vi "CSMsettings_ut_test.vi"(8 "Error In":errorcluster, 11 "CSMinfo in":T3={"Общие сведения"={"Регистрационный номер заказа"="", "Идентификация (шифр) образца"="", "IMEI образца"="", "НД, устанавливающий требования"="", "Методы испытаний (измерений)"="", "Дата начала испытаний"="", "Дата завершения испытаний"=""}, "Климатические условия внешней среды"={"Температура окружающего воздуха"="", "Относительная влажность воздуха"="", "Атмосферное давление"=""}, "Окно с настройками"={"Режим звонка связь"=0, "Напряжение источника"=0, "Условия окружающей среды"=0, "Номер образца"=0, "Источник питания"=0, "Номер испытания"=0, "Режим звонка тональный модем"=0, "Количество итераций TM"=100.0, "Аутентификация"=0, "Колличество повторов измерений"=1.0, "Сим карта"=0, "VISA adress of CMW500"="", "Input attenuation"=1.0, "Output attenuation"=1.0, "Call Release Type"=0, "GSM Band"=0, "BCCH Channel Number"=0.0, "TCH Channel Number"=0.0, "Codec"=0, "AWGN"=0, "snrRatioInDb"=0.0, "GSM Fading"=0, "UL C/I ratio"=0, "Use a custom network ID"=FALSE, "MCC (Mobile Country Code)"=0.0, "MNC (Mobile Network Code)"=0.0, "NCC (Network Color Code)"=0.0, "MNC digit count"=0, "BCC (Base station Color Code)"=0.0, "LAC (Location Area Code)"=0.0, "RAC (Routing Area Code)"=0.0, "Cell Identity"=0.0, "Override UE ID"=FALSE, "MCC (UE Mobile Country Code)"=0.0, "MNC (UE Mobile Network Code)"=0.0, "MSIN (Mobile Subscription ID)"=0.0, "InputScaleFactor"=0, "OutputScaleFactor"=0, "Post MSD wave file playback 3GPP  26.269 \nEU_DTMF_tones"=FALSE, "Scenario"=0, "AlAckBehavior"=0, "PSAP listens for PUSH"=FALSE, "BCCH Channel Power"=0.0, "TCH Channel Power"=0.0, "Setting Path"=path "", "Алгоритм дозвона"=0}} {"Окно с настройками"."Алгоритм дозвона" items=["Standart", "Recall"]; "Окно с настройками"."AlAckBehavior" items=["POSITIVE", "CLEAR_DOWN", "LOOP_BACK_MSD_PART"]; "Окно с настройками"."Scenario" items=["NORMAL", "NORMAL_IMMEDIATE_START", "TIMEOUT_T3", "ALLRV_REQ", "SUPPRESS_MSD", "SUPPRESS_ALACK", "SUPPRESS_SEND_MSD"]; "Окно с настройками"."OutputScaleFactor" items=["ONE", "QUARTER", "HALF", "TWO", "FOUR"]; "Окно с настройками"."InputScaleFactor" items=["ONE", "QUARTER", "HALF", "TWO", "FOUR"]; "Окно с настройками"."MNC digit count" items=["TWO", "THREE"]; "Окно с настройками"."UL C/I ratio" items=["Ci1Db", "Ci4Db", "Ci7Db", "Ci10Db", "Ci13Db", "Ci16Db"]; "Окно с настройками"."GSM Fading" items=["GsmFadingOff", "GsmEtsiTs103412DlFading", "GsmEtsiTs103412UlFading", "GsmEtsiTs103412DlUlFading"]; "Окно с настройками"."AWGN" items=["Off", "50MhzAwgn"]; "Окно с настройками"."Codec" items=["FRV2", "AMRH_GMSK_7K95", "AMRH_GMSK_7K40", "AMRH_GMSK_6K70", "AMRH_GMSK_5K90", "AMRH_GMSK_5K15", "AMRH_GMSK_4K75", "AMRF_GMSK_12K20", "AMRF_GMSK_10K20", "AMRF_GMSK_7K95", "AMRF_GMSK_7K40 ", "AMRF_GMSK_6K70", "AMRF_GMSK_5K90", "AMRF_GMSK_5K15", "AMRF_GMSK_4K75", "FRV1", "HRV1", "WAMR_GMSK_6K60", "WAMR_GMSK_8K85", "WAMR_GMSK_12K65"]; "Окно с настройками"."GSM Band" items=["GSM450", "GSM850", "GSM900", "GSM1800", "GSM1900"]; "Окно с настройками"."Call Release Type" items=["NormalRelease", "CallInterruption"]; "Окно с настройками"."Сим карта" items=["SIM", "eSIM"]; "Окно с настройками"."Колличество повторов измерений" min=1.0 max=100.0 format="%#_3g"; "Окно с настройками"."Аутентификация" items=["On", "Off"]; "Окно с настройками"."Режим звонка тональный модем" items=["Автоматически (AT) GEMALTO", "Автоматически (AT) SIMCOM", "Автоматически (AT) SIMCOM SIM7600E-H", "Автоматически (AT) TELIT", "Автоматически (AT) PROGRESS", "Автоматически (AT) PROGRESS GREEN", "Автоматически (AT) PROGRESS BLUE", "Автоматически (реле)", "Вручную"]; "Окно с настройками"."Номер испытания" items=["1", "2", "3"]; "Окно с настройками"."Источник питания" items=["Не используется", "IT6332A"]; "Окно с настройками"."Номер образца" items=["1", "2", "3"]; "Окно с настройками"."Условия окружающей среды" items=["UnormTnorm", "UminTmin", "UmaxTmin", "UminTmax", "UmaxTmax", "TypeA", "TypeB"]; "Окно с настройками"."Напряжение источника" items=["12", "24"]; "Окно с настройками"."Режим звонка связь" items=["Автоматически (AT) GEMALTO", "Автоматически (AT) SIMCOM", "Автоматически (AT) SIMCOM SIM7600E-H", "Автоматически (AT) TELIT", "Автоматически (AT) PROGRESS", "Автоматически (AT) PROGRESS GREEN", "Автоматически (AT) PROGRESS BLUE", "Автоматически (реле)", "Вручную"]}) -> (0 "Error Out":errorcluster, 3 "CSMinfo out":T3={"Общие сведения"={"Регистрационный номер заказа"="", "Идентификация (шифр) образца"="", "IMEI образца"="", "НД, устанавливающий требования"="", "Методы испытаний (измерений)"="", "Дата начала испытаний"="", "Дата завершения испытаний"=""}, "Климатические условия внешней среды"={"Температура окружающего воздуха"="", "Относительная влажность воздуха"="", "Атмосферное давление"=""}, "Окно с настройками"={"Режим звонка связь"=0, "Напряжение источника"=0, "Условия окружающей среды"=0, "Номер образца"=0, "Источник питания"=0, "Номер испытания"=0, "Режим звонка тональный модем"=0, "Количество итераций TM"=0.0, "Аутентификация"=0, "Колличество повторов измерений"=1.0, "Сим карта"=0, "VISA adress of CMW500"="", "Input attenuation"=1.0, "Output attenuation"=1.0, "Call Release Type"=0, "GSM Band"=0, "BCCH Channel Number"=0.0, "TCH Channel Number"=0.0, "Codec"=0, "AWGN"=0, "snrRatioInDb"=0.0, "GSM Fading"=0, "UL C/I ratio"=0, "Use a custom network ID"=FALSE, "MCC (Mobile Country Code)"=0.0, "MNC (Mobile Network Code)"=0.0, "NCC (Network Color Code)"=0.0, "MNC digit count"=0, "BCC (Base station Color Code)"=0.0, "LAC (Location Area Code)"=0.0, "RAC (Routing Area Code)"=0.0, "Cell Identity"=0.0, "Override UE ID"=FALSE, "MCC (UE Mobile Country Code)"=0.0, "MNC (UE Mobile Network Code)"=0.0, "MSIN (Mobile Subscription ID)"=0.0, "InputScaleFactor"=0, "OutputScaleFactor"=0, "Post MSD wave file playback 3GPP  26.269 \nEU_DTMF_tones"=FALSE, "Scenario"=0, "AlAckBehavior"=0, "PSAP listens for PUSH"=FALSE, "BCCH Channel Power"=0.0, "TCH Channel Power"=0.0, "Setting Path"=path "", "Алгоритм дозвона"=0}} {"Окно с настройками"."Алгоритм дозвона" items=["Standart", "Recall"]; "Окно с настройками"."AlAckBehavior" items=["POSITIVE", "CLEAR_DOWN", "LOOP_BACK_MSD_PART"]; "Окно с настройками"."Scenario" items=["NORMAL", "NORMAL_IMMEDIATE_START", "TIMEOUT_T3", "ALLRV_REQ", "SUPPRESS_MSD", "SUPPRESS_ALACK", "SUPPRESS_SEND_MSD"]; "Окно с настройками"."OutputScaleFactor" items=["ONE", "QUARTER", "HALF", "TWO", "FOUR"]; "Окно с настройками"."InputScaleFactor" items=["ONE", "QUARTER", "HALF", "TWO", "FOUR"]; "Окно с настройками"."MNC digit count" items=["TWO", "THREE"]; "Окно с настройками"."UL C/I ratio" items=["Ci1Db", "Ci4Db", "Ci7Db", "Ci10Db", "Ci13Db", "Ci16Db"]; "Окно с настройками"."GSM Fading" items=["GsmFadingOff", "GsmEtsiTs103412DlFading", "GsmEtsiTs103412UlFading", "GsmEtsiTs103412DlUlFading"]; "Окно с настройками"."AWGN" items=["Off", "50MhzAwgn"]; "Окно с настройками"."Codec" items=["FRV2", "AMRH_GMSK_7K95", "AMRH_GMSK_7K40", "AMRH_GMSK_6K70", "AMRH_GMSK_5K90", "AMRH_GMSK_5K15", "AMRH_GMSK_4K75", "AMRF_GMSK_12K20", "AMRF_GMSK_10K20", "AMRF_GMSK_7K95", "AMRF_GMSK_7K40 ", "AMRF_GMSK_6K70", "AMRF_GMSK_5K90", "AMRF_GMSK_5K15", "AMRF_GMSK_4K75", "FRV1", "HRV1", "WAMR_GMSK_6K60", "WAMR_GMSK_8K85", "WAMR_GMSK_12K65"]; "Окно с настройками"."GSM Band" items=["GSM450", "GSM850", "GSM900", "GSM1800", "GSM1900"]; "Окно с настройками"."Call Release Type" items=["NormalRelease", "CallInterruption"]; "Окно с настройками"."Сим карта" items=["SIM", "eSIM"]; "Окно с настройками"."Колличество повторов измерений" min=1.0 max=100.0 format="%#_3g"; "Окно с настройками"."Аутентификация" items=["On", "Off"]; "Окно с настройками"."Режим звонка тональный модем" items=["Автоматически (AT) GEMALTO", "Автоматически (AT) SIMCOM", "Автоматически (AT) SIMCOM SIM7600E-H", "Автоматически (AT) TELIT", "Автоматически (AT) PROGRESS", "Автоматически (AT) PROGRESS GREEN", "Автоматически (AT) PROGRESS BLUE", "Автоматически (реле)", "Вручную"]; "Окно с настройками"."Номер испытания" items=["1", "2", "3"]; "Окно с настройками"."Источник питания" items=["Не используется", "IT6332A"]; "Окно с настройками"."Номер образца" items=["1", "2", "3"]; "Окно с настройками"."Условия окружающей среды" items=["UnormTnorm", "UminTmin", "UmaxTmin", "UminTmax", "UmaxTmax", "TypeA", "TypeB"]; "Окно с настройками"."Напряжение источника" items=["12", "24"]; "Окно с настройками"."Режим звонка связь" items=["Автоматически (AT) GEMALTO", "Автоматически (AT) SIMCOM", "Автоматически (AT) SIMCOM SIM7600E-H", "Автоматически (AT) TELIT", "Автоматически (AT) PROGRESS", "Автоматически (AT) PROGRESS GREEN", "Автоматически (AT) PROGRESS BLUE", "Автоматически (реле)", "Вручную"]})   [LabVIEW 2018]
uses:
  CSMinfo.ctl
  MOKO_LabViewLibrary/MokoSTM/MokoClassicUtilitySTM/MCUS_STM.ctl
  MOKO_LabViewLibrary/MokoSTM/MokoClassicUtilitySTM/MCUS_ITEM.ctl
  <vilib>/addons/_JKI.lib/Serialization/JSON/JKI JSON Serialization.lvlib
panel:
  in  "Reset":bool
  in  "Open":bool
  in  "Save":bool
  in  "Setting Path":path
  in  "Применить":bool
  in  "Общие настройки/Настройки модема":T1(tab)
  in  "Алгоритм дозвона":u16(ring) items=["Standart", "Recall"]
  in  "Сим карта":u16(ring) items=["SIM", "eSIM"]
  in  "Количество повторов измерений":dbl=1.0
  in  "Аунтетификация":u16(ring) items=["On", "Off"]
  in  "Количество итераций TM":dbl=100.0
  in  "Условия окружающей среды":u16(ring) items=["UnormTnorm", "UminTmin", "UmaxTmin", "UminTmax", "UmaxTmax", "TypeA", "TypeB"]
  in  "Режим звонка тональный модем":u16(ring) items=["Автоматически (AT) GEMALTO", "Автоматически (AT) SIMCOM", "Автоматически (AT) SIMCOM SIM7600E-H", "Автоматически (AT) TELIT", "Автоматически (AT) PROGRESS", "Автоматически (AT) PROGRESS GREEN", "Автоматически (AT) PROGRESS BLUE", "Автоматически (реле)", "Вручную"]
  in  "Номер испытания":u16(ring) items=["1", "2", "3"]
  in  "Источник питания":u16(ring) items=["Не используется", "IT6332A"]
  in  "Напряжение источника":u16(ring) items=["12", "24"]
  in  "Номер образца":u16(ring) items=["1", "2", "3"]
  in  "Режим звонка связь":u16(ring) items=["Автоматически (AT) GEMALTO", "Автоматически (AT) SIMCOM", "Автоматически (AT) SIMCOM SIM7600E-H", "Автоматически (AT) TELIT", "Автоматически (AT) PROGRESS", "Автоматически (AT) PROGRESS GREEN", "Автоматически (AT) PROGRESS BLUE", "Автоматически (реле)", "Вручную"]
  in  "Настройки модема по умолчанию":enum32{"CMW500", "GSM", "PSAP"}(tab)
  in  "VISA adress of CMW500":string="TCPIP0::169.254.98.10::inst0::INSTR"
  in  "Input attenuation":dbl=1.0
  in  "Output attenuation":dbl=100.0
  in  "GSM":T2(tab)
  in  "BCCH Channel Power":dbl=1.0
  in  "TCH Channel Power":dbl=1.0
  in  "GSM Band":u16(ring) items=["GSM450", "GSM850", "GSM900", "GSM1800", "GSM1900"]
  in  "BCCH Channel Number":dbl=1.0
  in  "TCH Channel number":dbl=1.0
  in  "Codec":u16(ring) items=["FRV2", "AMRH_GMSK_7K95", "AMRH_GMSK_7K40", "AMRH_GMSK_6K70", "AMRH_GMSK_5K90", "AMRH_GMSK_5K15", "AMRH_GMSK_4K75", "AMRF_GMSK_12K20", "AMRF_GMSK_10K20", "AMRF_GMSK_7K95", "AMRF_GMSK_7K40 ", "AMRF_GMSK_6K70", "AMRF_GMSK_5K90", "AMRF_GMSK_5K15", "AMRF_GMSK_4K75", "FRV1", "HRV1", "WAMR_GMSK_6K60", "WAMR_GMSK_8K85", "WAMR_GMSK_12K65"]
  in  "AWGN":u16(ring) items=["Off", "50MhzAwgn"]
  in  "snrRatioInDb":dbl=1.0
  in  "GSM Fading":u16(ring) items=["GsmFadingOff", "GsmEtsiTs103412DlFading", "GsmEtsiTs103412UlFading", "GsmEtsiTs103412DlUlFading"]
  in  "UL C/I ratio":u16(ring) items=["Ci1Db", "Ci4Db", "Ci7Db", "Ci10Db", "Ci13Db", "Ci16Db"]
  in  "MCC (Mobile Country Code)":dbl=1.0
  in  "Use a custom network ID":bool
  in  "MNC (Mobile Network Code)":dbl=1.0
  in  "MNC digit count":u16(ring) items=["TWO", "THREE"]
  in  "BCC (Base station Color Code)":dbl=1.0
  in  "NCC (Network Color Code)":dbl=1.0
  in  "RAC (Routing Area Code)":dbl=1.0
  in  "LAC (Location Area Code)":dbl=1.0
  in  "Cell Identity":dbl=1.0
  in  "Override UE ID":bool
  in  "MNC (UE Mobile Network Code)":dbl=1.0
  in  "MCC (UE Mobile Country Code)":dbl=1.0
  in  "MSIN (Mobile Subscription ID)":dbl=1.0 format="%#_10g"
  in  "Call Release Type":u16(ring) items=["NormalRelease", "CallInterruption"]
  in  "OutputScaleFactor":u16(ring) items=["ONE", "QUARTER", "HALF", "TWO", "FOUR"]
  in  "PSAP listens for PUSH":bool
  in  "AlAckBehavior":u16(ring) items=["POSITIVE", "CLEAR_DOWN", "LOOP_BACK_MSD_PART"]
  in  "Scenario":u16(ring) items=["NORMAL", "NORMAL_IMMEDIATE_START", "TIMEOUT_T3", "ALLRV_REQ", "SUPPRESS_MSD", "SUPPRESS_ALACK", "SUPPRESS_SEND_MSD"]
  in  "InputScaleFactor":u16(ring) items=["ONE", "QUARTER", "HALF", "TWO", "FOUR"]
  in  "Post MSD wave file playback 3GPP  26.269 EU_DTMF_tones":bool
  # "0,4\n0,6\n1\n1,5\n1,6\n2,5\n4"
  # "kPa\nbar\nkgf/cm2\nMPa"
  # "1. Общие настройки"
  # "Номер образца:"
  # "Номер испытания:"
  # "Режим измерения:"
  # "Источник питания:"
  # "Напряжение источника питания, B:"
  # "2. Настройки связи"
  # "Режим звонка:"
  # "Аунтетификация:"
  # "Сим карта:"
  # "Количество повторов измерений:"
  # "3. Настройки тонального модема"
  # "Режим звонка:"
  # "Алгоритм дозвона:"
  # "Количество итераций Tonal:"
  # "VISA adress of CMW500:"
  # "Input attenuation:"
  # "Output attenuation:"
  # "GSM Band:"
  # "BCCH Channel Power"
  # "TCH Channel Power"
  # "BCCH Channel Number"
  # "TCH Channel number"
  # "Codec"
  # "8.6.6"
  # "AWGN"
  # "snrRatioInDb"
  # "GSM Fading"
  # "UL C/I ratio"
  # "MCC (Mobile Country Code)"
  # "MNC (Mobile Network Code)"
  # "MNC digit count"
  # "NCC (Network Color Code)"
  # "BCC (Base station Color Code)"
  # "LAC (Location Area Code)"
  # "RAC (Routing Area Code)"
  # "Cell Identity"
  # "MCC (UE Mobile Country Code)"
  # "MNC (UE Mobile Network Code)"
  # "MSIN (Mobile Subscription ID)"
  # "Call Release Type:"
  # "8.6.6"
  # "InputScaleFactor"
  # "OutputScaleFactor"
  # "8.6.7"
  # "8.6.8 (Use parameter NORMAL_IMMEDIATE_START)"
  # "Scenario"
  # "8.6.9 (Use parameter LOOP_BACK_MSD_PART)"
  # "AlAckBehavior"
  # "1. Общие настройки"
  # "Настройки модема по умолчанию"
  # "CMW500"
  # "PSAP"
  # "8.6.6"
  # "8.6.7"
  # "GSM"
  # "2. Настройки связи"
  # "8.6.8 (Use parameter NORMAL_IMMEDIATE_START)"
  # "8.6.9 (Use parameter LOOP_BACK_MSD_PART)"
  # "8.6.6"
  # "3. Настройки тонального модема"
  # "1. Общие настройки"
  # "Настройки модема по умолчанию"
  # "CMW500"
  # "PSAP"
  # "8.6.6"
  # "8.6.7"
  # "GSM"
  # "2. Настройки связи"
  # "8.6.8 (Use parameter NORMAL_IMMEDIATE_START)"
  # "8.6.9 (Use parameter LOOP_BACK_MSD_PART)"
  # "8.6.6"
  # "3. Настройки тонального модема"
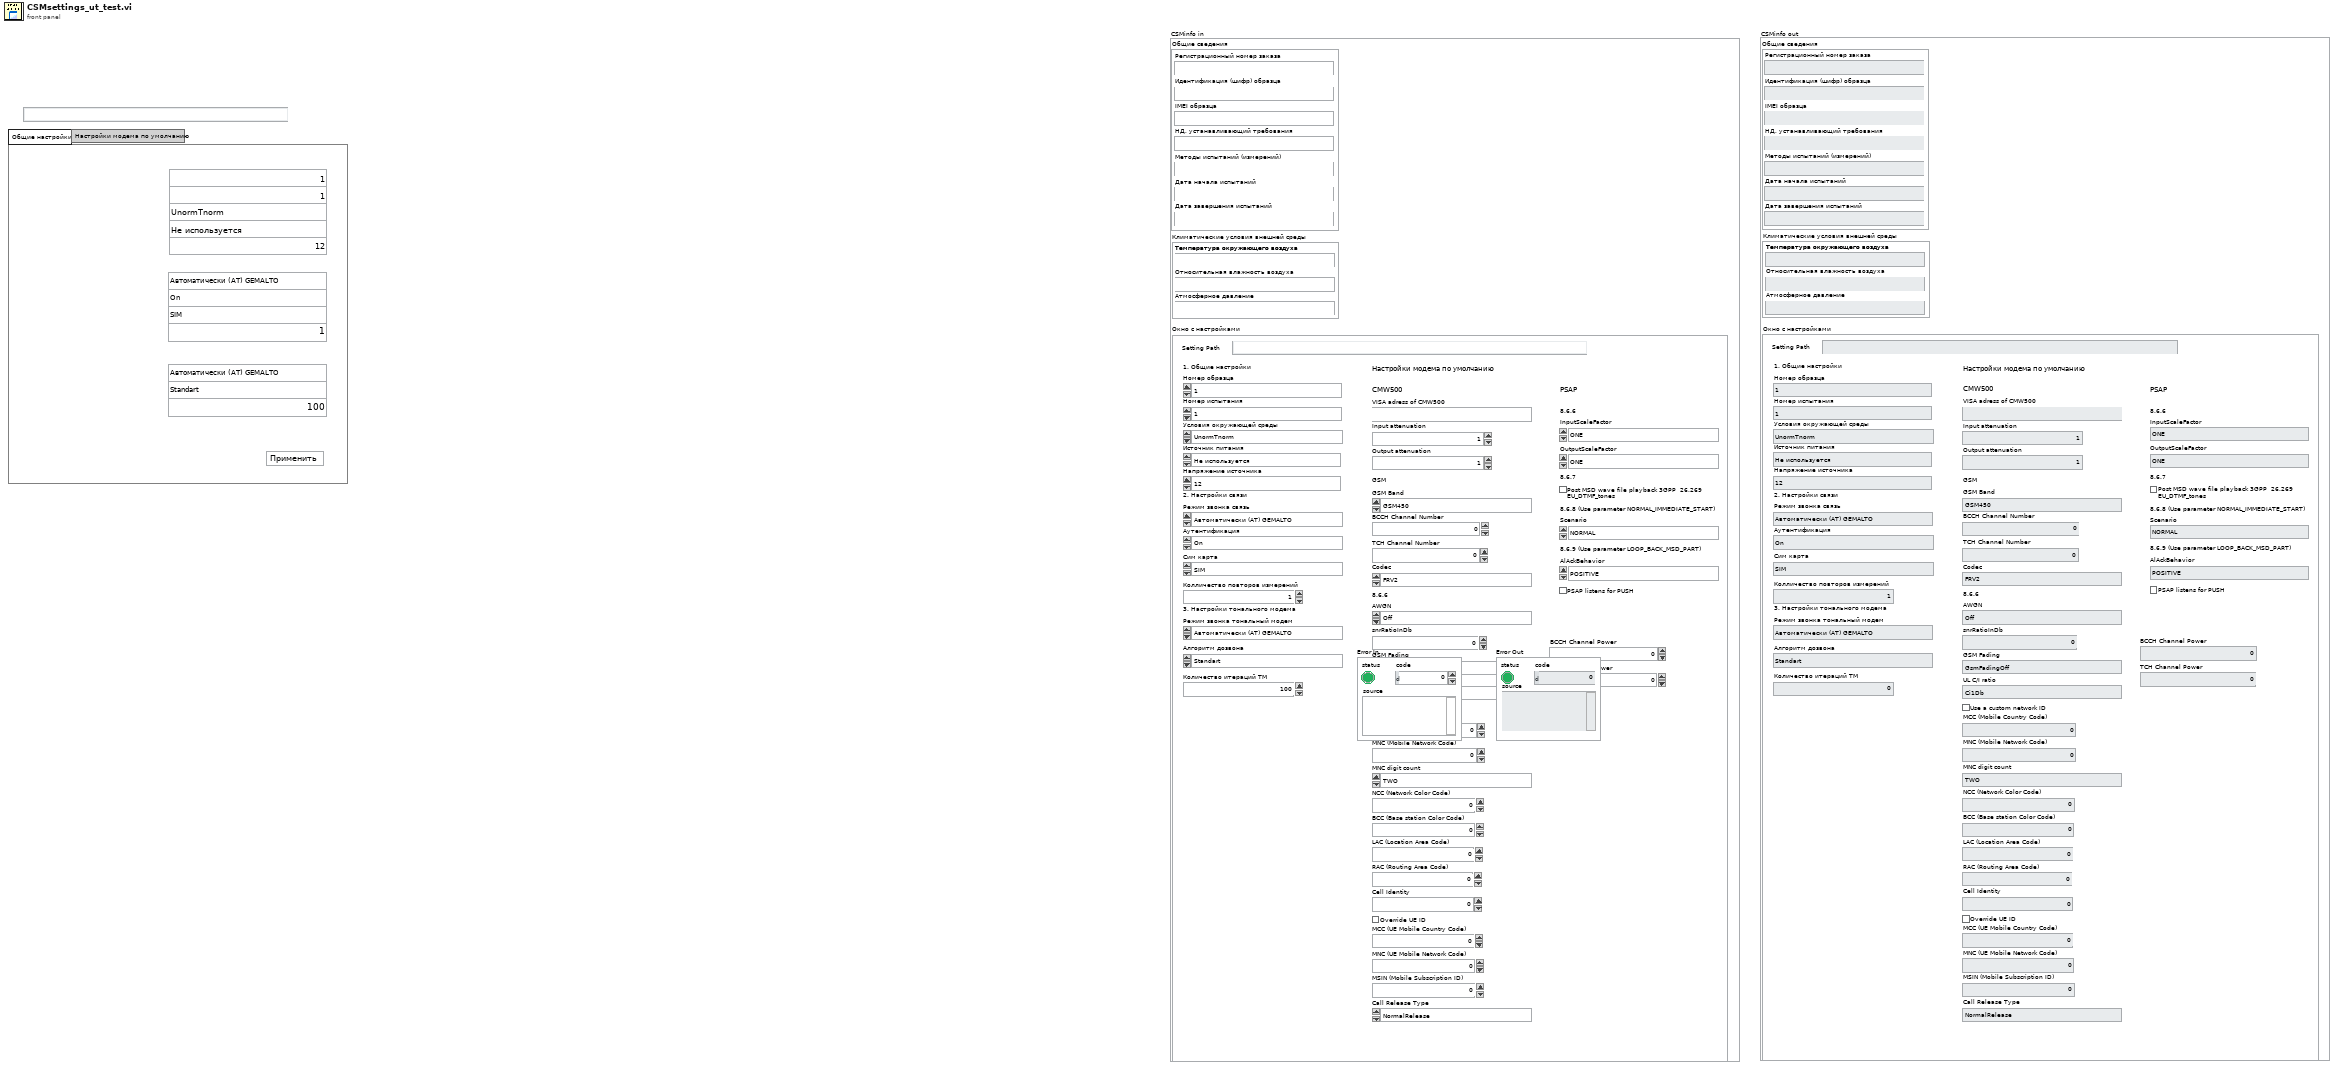
[diagram p1: front panel]
types:
  T1 = enum32{"Общие настройки", "Настройки модема по умолчанию"}
  T2 = enum32{"GSM Band/AWGN", "Custom network ID", "Call Release Type"}
  T3 = typedef "CSMinfo.ctl" = cluster{"Общие сведения":cluster{"Регистрационный номер заказа":string, "Идентификация (шифр) образца":string, "IMEI образца":string, "НД, устанавливающий требования":string, "Методы испытаний (измерений)":string, "Дата начала испытаний":string, "Дата завершения испытаний":string}, "Климатические условия внешней среды":cluster{"Температура окружающего воздуха":string, "Относительная влажность воздуха":string, "Атмосферное давление":string}, "Окно с настройками":cluster{"Режим звонка связь":u16, "Напряжение источника":u16, "Условия окружающей среды":u16, "Номер образца":u16, "Источник питания":u16, "Номер испытания":u16, "Режим звонка тональный модем":u16, "Количество итераций TM":dbl, "Аутентификация":u16, "Колличество повторов измерений":dbl, "Сим карта":u16, "VISA adress of CMW500":string, "Input attenuation":dbl, "Output attenuation":dbl, "Call Release Type":u16, "GSM Band":u16, "BCCH Channel Number":dbl, "TCH Channel Number":dbl, "Codec":u16, "AWGN":u16, "snrRatioInDb":dbl, "GSM Fading":u16, "UL C/I ratio":u16, "Use a custom network ID":bool, "MCC (Mobile Country Code)":dbl, "MNC (Mobile Network Code)":dbl, "NCC (Network Color Code)":dbl, "MNC digit count":u16, "BCC (Base station Color Code)":dbl, "LAC (Location Area Code)":dbl, "RAC (Routing Area Code)":dbl, "Cell Identity":dbl, "Override UE ID":bool, "MCC (UE Mobile Country Code)":dbl, "MNC (UE Mobile Network Code)":dbl, "MSIN (Mobile Subscription ID)":dbl, "InputScaleFactor":u16, "OutputScaleFactor":u16, "Post MSD wave file playback 3GPP  26.269 \nEU_DTMF_tones":bool, "Scenario":u16, "AlAckBehavior":u16, "PSAP listens for PUSH":bool, "BCCH Channel Power":dbl, "TCH Channel Power":dbl, "Setting Path":path, "Алгоритм дозвона":u16}}
  T4 = typedef "MCUS_STM.ctl" = cluster{"main stm":T5, "data":string}
  T5 = typedef "MCUS_ITEM.ctl" = enum16{"idle", "_____ main_____ ", "Init", "Stop", "Apply values", "Save", "Open", "Reset"}
  T6 = cluster{"Режим звонка связь":u16, "Напряжение источника":u16, "Условия окружающей среды":u16, "Номер образца":u16, "Источник питания":u16, "Номер испытания":u16, "Режим звонка тональный модем":u16, "Количество итераций TM":dbl, "Аутентификация":u16, "Колличество повторов измерений":dbl, "Сим карта":u16, "VISA adress of CMW500":string, "Input attenuation":dbl, "Output attenuation":dbl, "Call Release Type":u16, "GSM Band":u16, "BCCH Channel Number":dbl, "TCH Channel Number":dbl, "Codec":u16, "AWGN":u16, "snrRatioInDb":dbl, "GSM Fading":u16, "UL C/I ratio":u16, "Use a custom network ID":bool, "MCC (Mobile Country Code)":dbl, "MNC (Mobile Network Code)":dbl, "NCC (Network Color Code)":dbl, "MNC digit count":u16, "BCC (Base station Color Code)":dbl, "LAC (Location Area Code)":dbl, "RAC (Routing Area Code)":dbl, "Cell Identity":dbl, "Override UE ID":bool, "MCC (UE Mobile Country Code)":dbl, "MNC (UE Mobile Network Code)":dbl, "MSIN (Mobile Subscription ID)":dbl, "InputScaleFactor":u16, "OutputScaleFactor":u16, "Post MSD wave file playback 3GPP  26.269 \nEU_DTMF_tones":bool, "Scenario":u16, "AlAckBehavior":u16, "PSAP listens for PUSH":bool, "BCCH Channel Power":dbl, "TCH Channel Power":dbl, "Setting Path":path, "Алгоритм дозвона":u16}
  T7 = enum16{"open", "replace", "create", "open or create", "replace or create", "replace or create with confirmation"}
  T8 = typedef "LVStringsAndValuesArrayTypeDef_U16.ctl" = cluster{"String":string, "Value":u16}[]
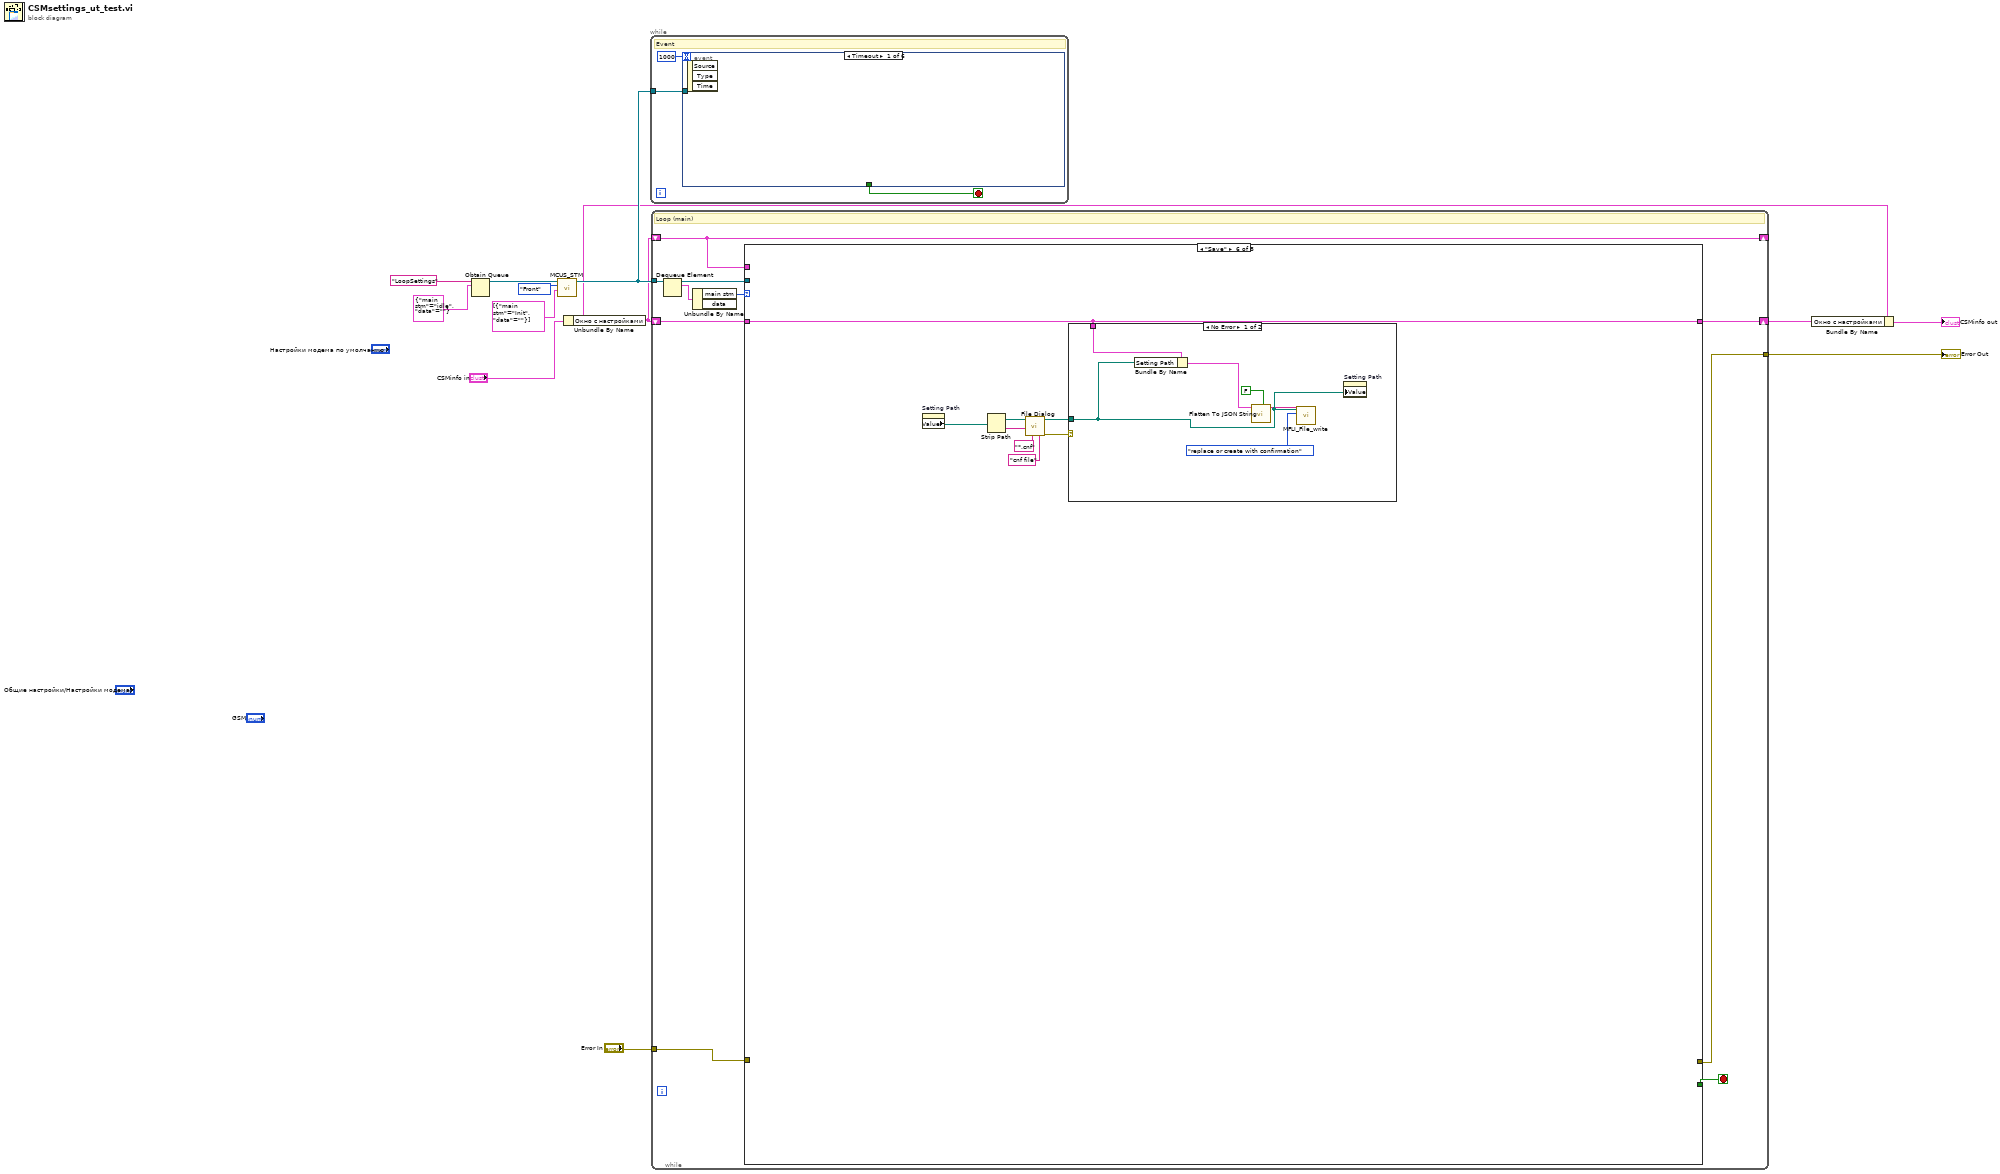
[diagram p0: block diagram]
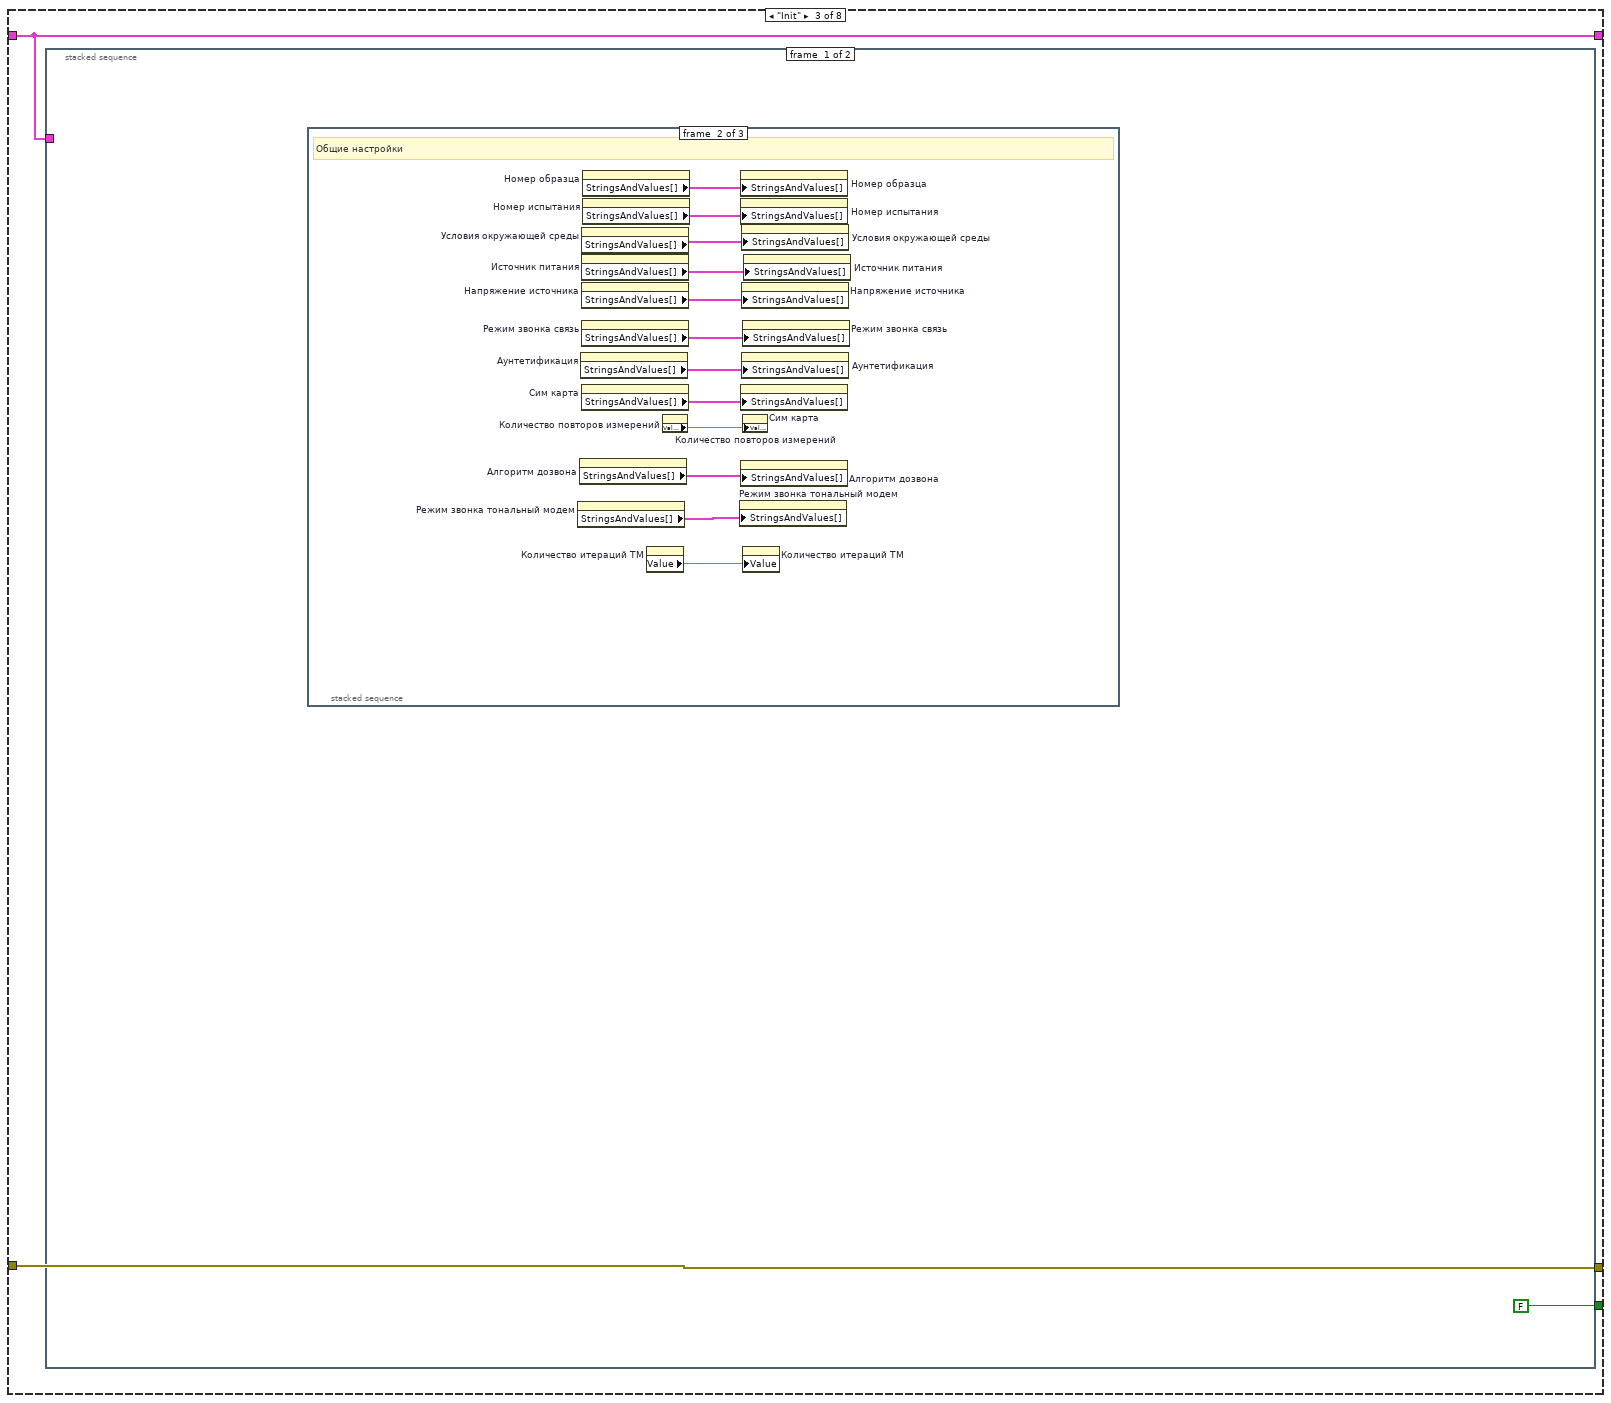
[diagram p4: hidden frame]
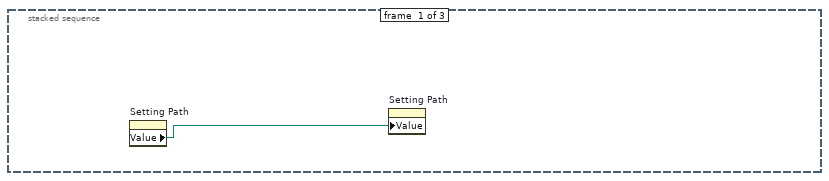
[diagram p5: hidden frame]
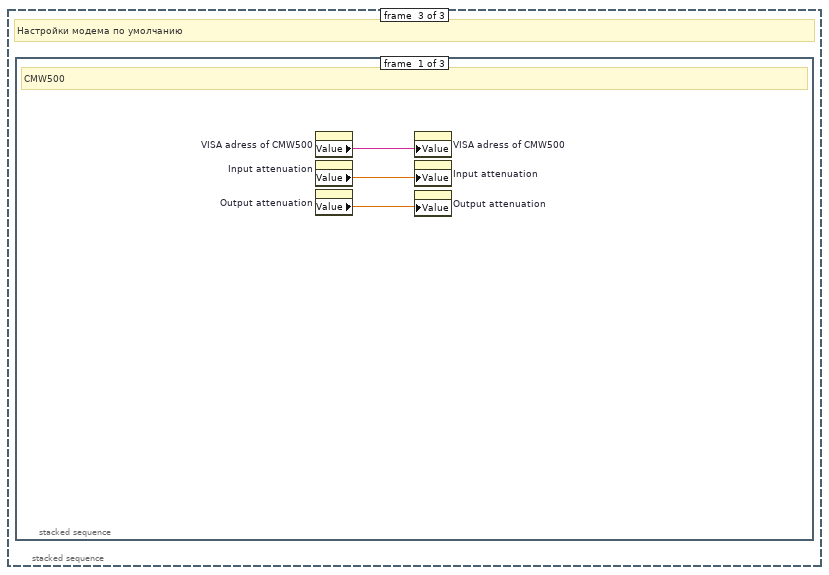
[diagram p6: hidden frame]
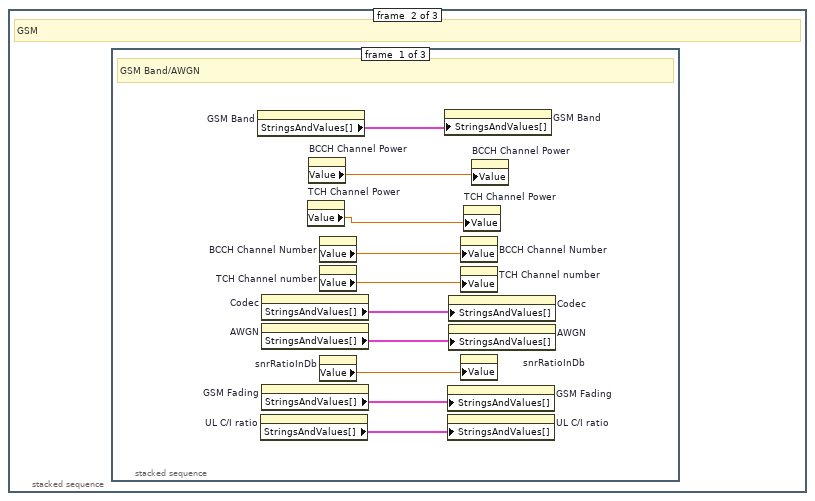
[diagram p7: hidden frame]
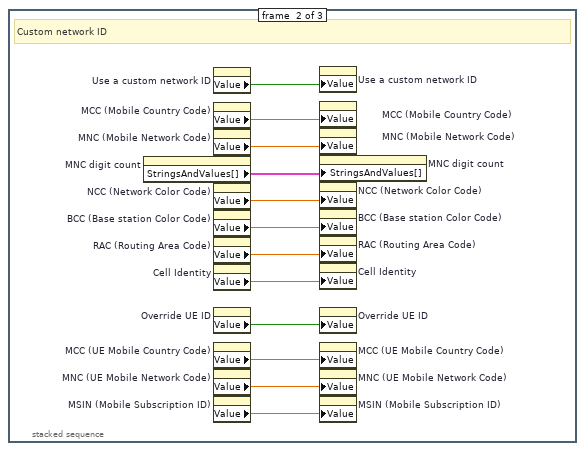
[diagram p8: hidden frame]
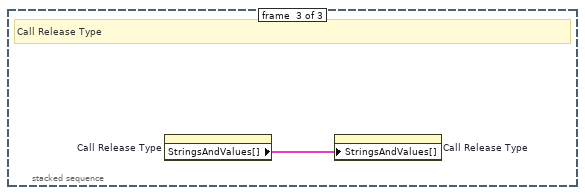
[diagram p9: hidden frame]
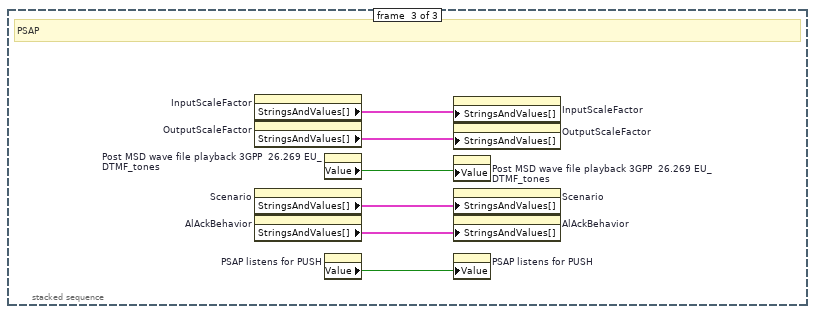
[diagram p10: hidden frame]
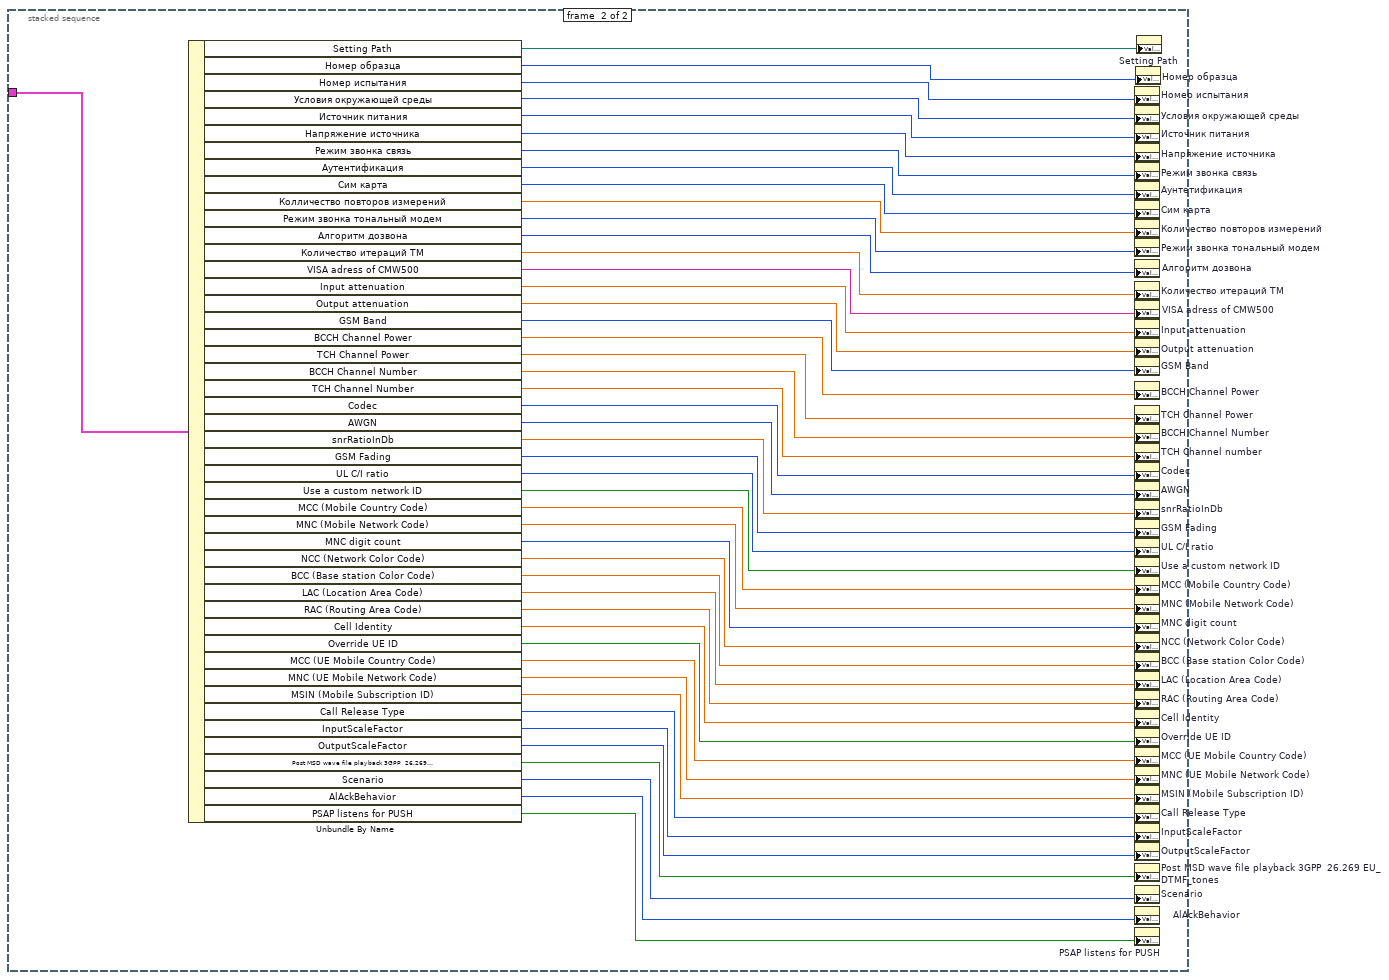
[diagram p11: hidden frame]
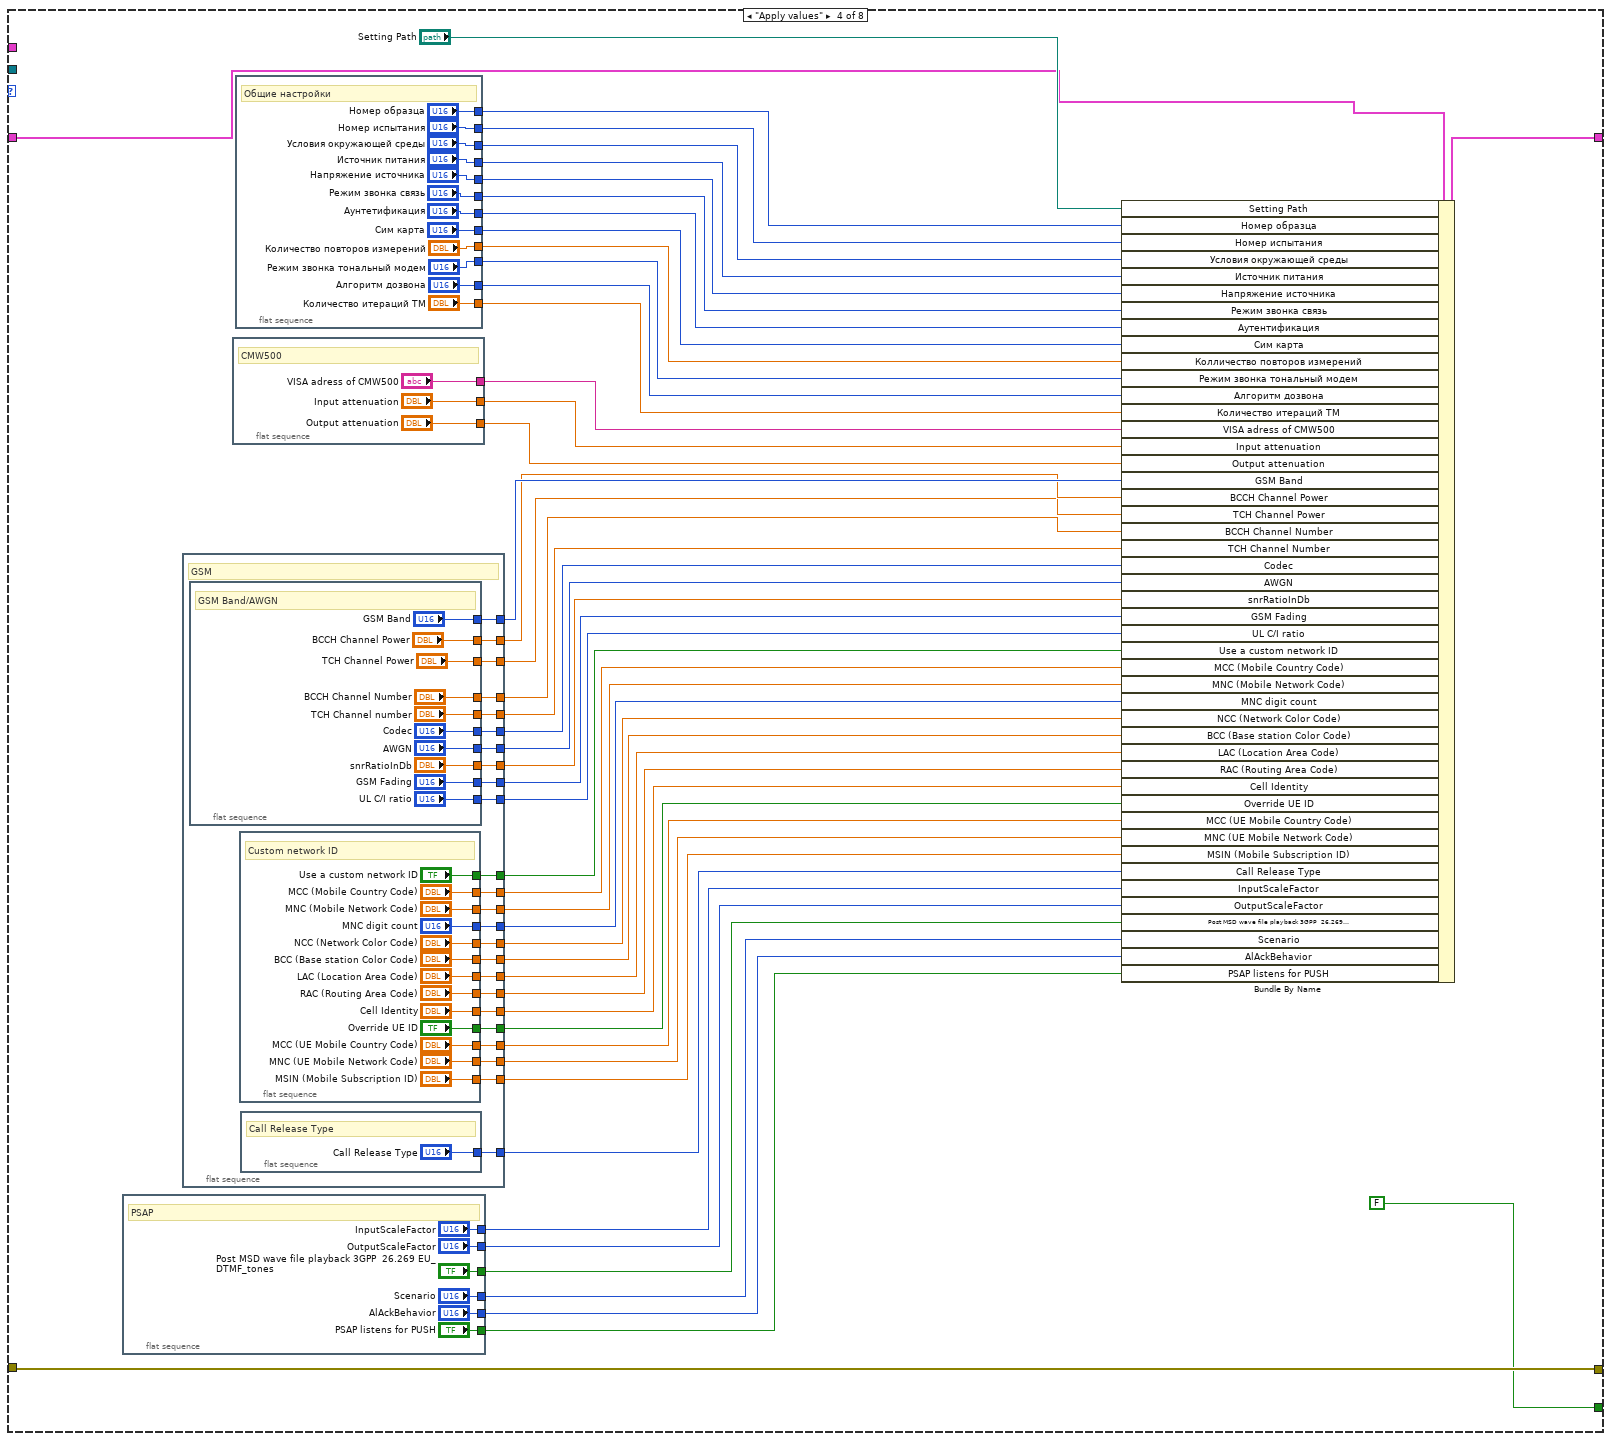
[diagram p12: hidden frame]
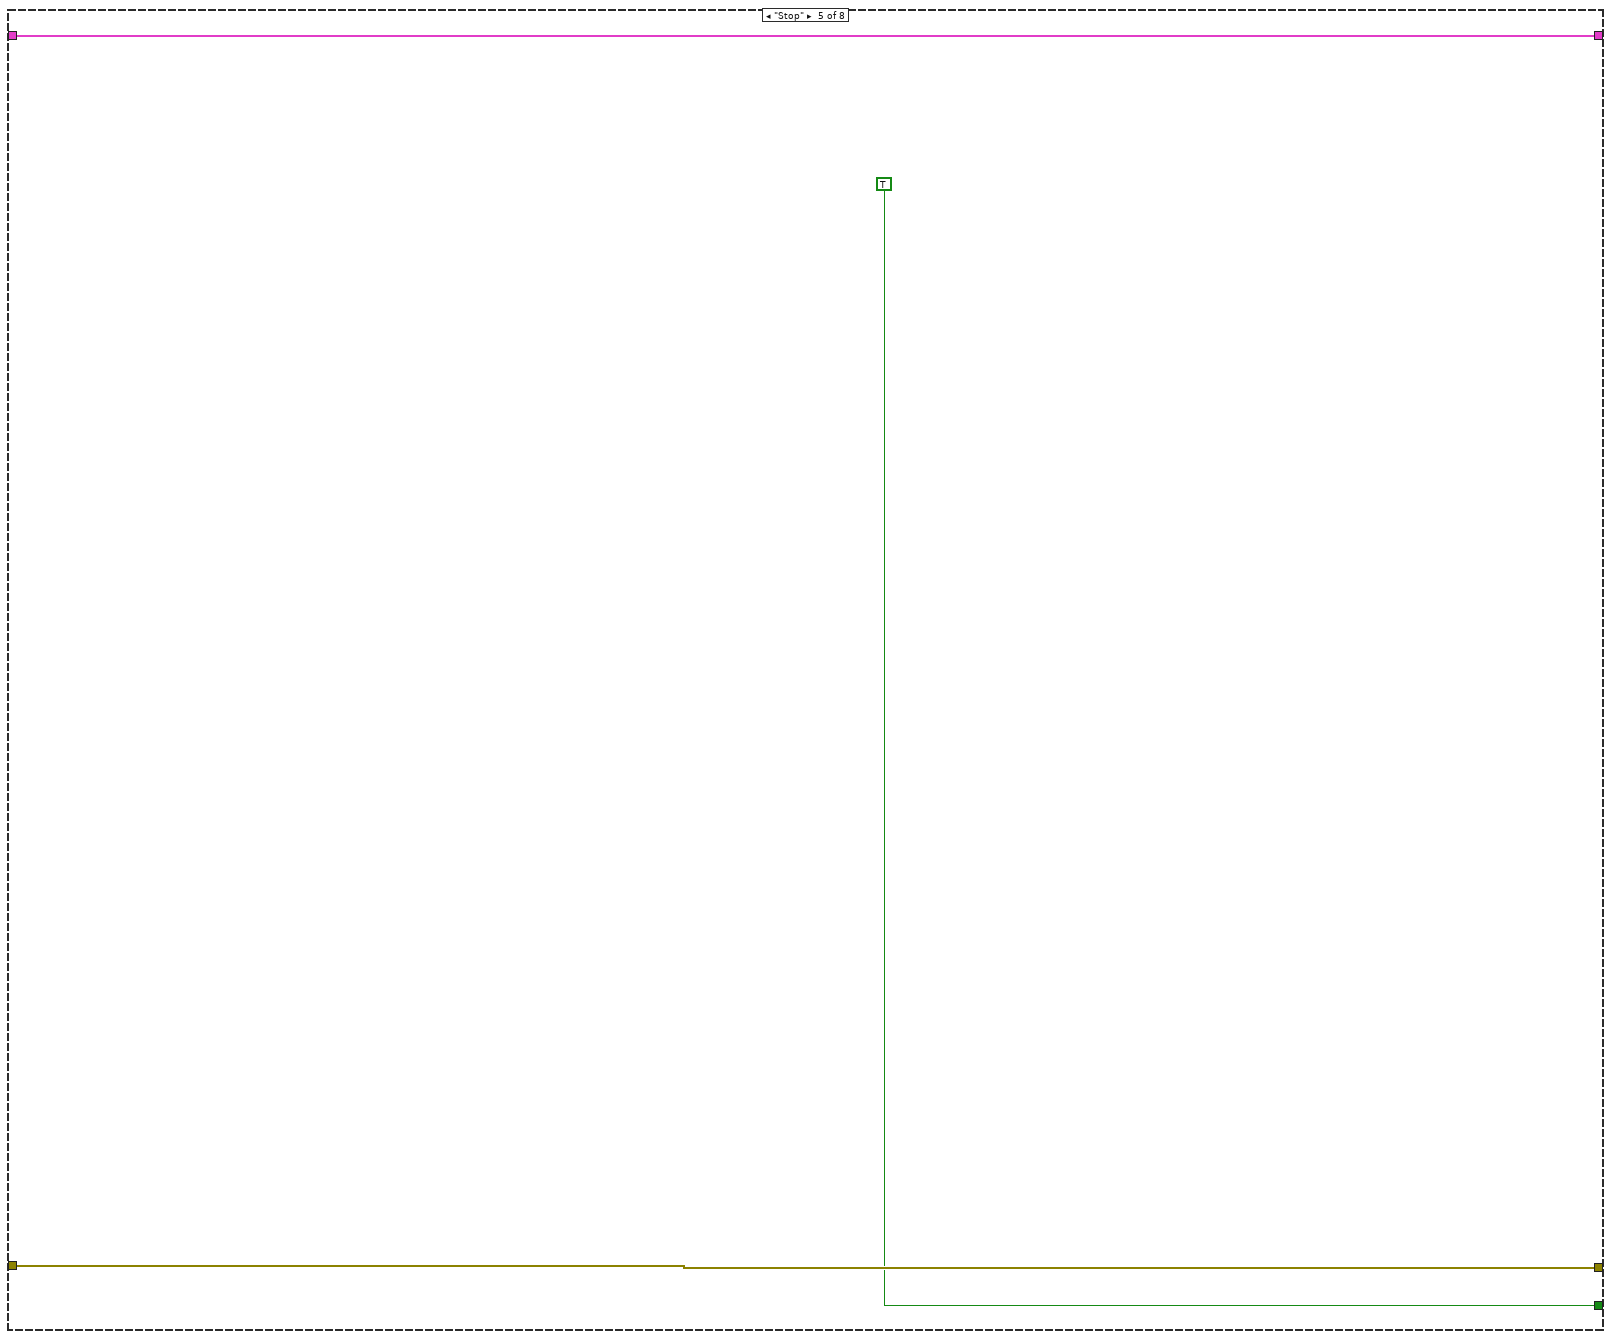
[diagram p13: hidden frame]
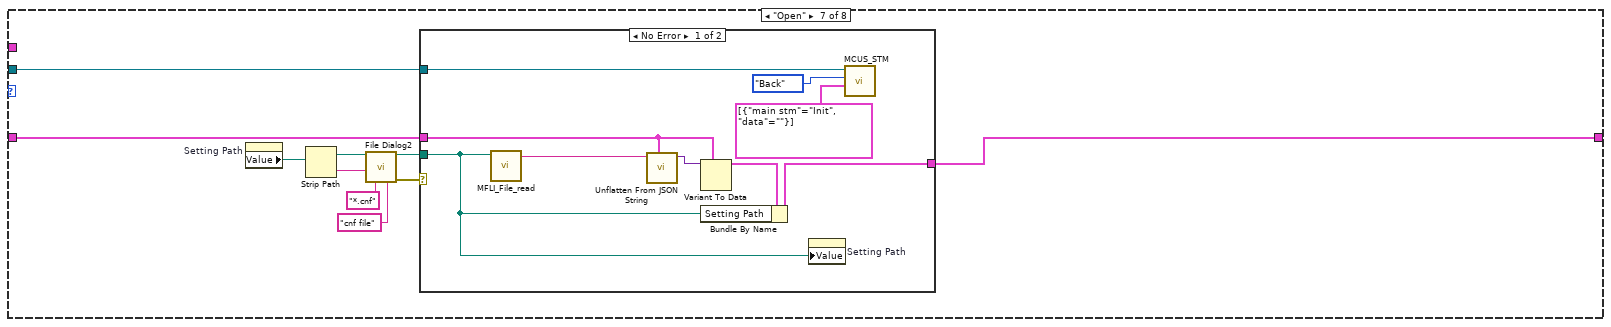
[diagram p15: hidden frame]
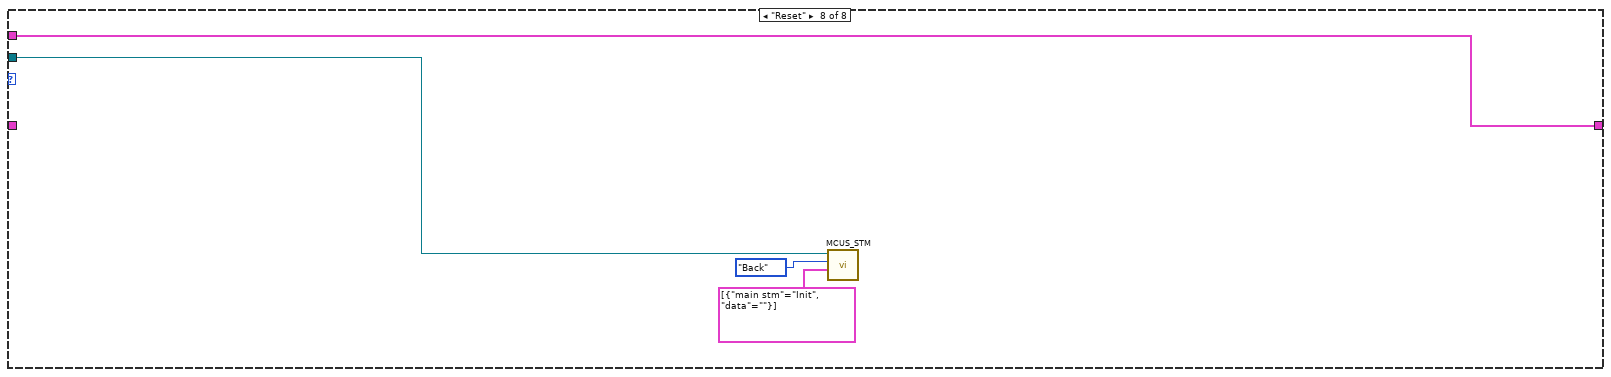
[diagram p17: hidden frame]
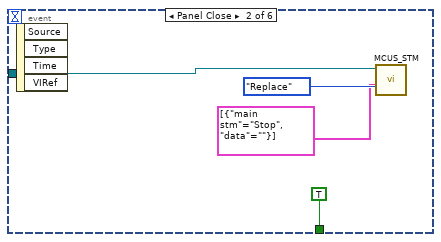
[diagram p18: hidden frame]
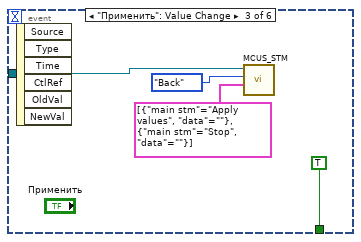
[diagram p19: hidden frame]
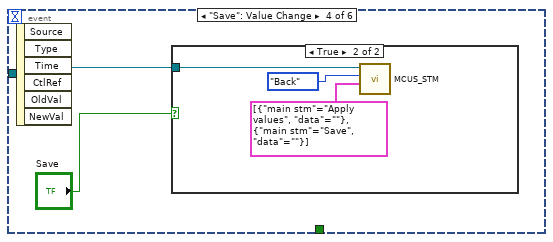
[diagram p20: hidden frame]
diagram:
  n1 = Obtain Queue(name (unnamed)="LoopSettings", element data type=T4 {"main stm"=enum."idle", "data"=""} ("MOKO_NMEA")) -> (queue out=w12:refnum<queue>)  [unwired: 3 in, 2 out]
  n2 = call "MCUS_STM.vi"("StateMachineSteps"=T4[] [{"main stm"=enum."Init", "data"=""}], "FNs"=enum16{"Back", "Front", "Replace"}."Front", "Queue in"=w12) -> ("Queue out"=w7:refnum<queue>)  [unwired: 7 in, 1 out]
  n3 = Unbundle By Name("CSMinfo in") -> ("Окно с настройками"=w4:T6)
  n4 = while {
    tunnel: w7 -> [w13]
    stop <- w15 stop-if-true
    # "Event"
    n5 = event shown="[0] Timeout" {
      selector: _ -> [_ _ _ _ _ _]
      dyn-events: _ -> [_ _ _ _ _ _]
      timeout: 1000 -> [_ _ _ _ _ _]
      tunnel: [_ TRUE TRUE _ _ _] -> w15
      tunnel: w13 -> [_ w16 w21 w25 w30 w35]
      event Timeout {
        n6 = event-data() -> ()  [unwired: 1 in, 3 out]
      }
      event Panel Close {
        n7 = event-data() -> ()  [unwired: 1 in, 4 out]
        n8 = call "MCUS_STM.vi"("StateMachineSteps"=T4[] [{"main stm"=enum."Stop", "data"=""}], "FNs"=enum16{"Back", "Front", "Replace"}."Replace", "Queue in"=w16) -> ()  [unwired: 7 in, 2 out]
      }
      event "Применить": Value Change {
        n9 = event-data() -> ()  [unwired: 1 in, 6 out]
        n10 = call "MCUS_STM.vi"("StateMachineSteps"=T4[] [{"main stm"=enum."Apply values", "data"=""}, {"main stm"=enum."Stop", "data"=""}], "FNs"=enum16{"Back", "Front", "Replace"}."Back", "Queue in"=w21) -> ()  [unwired: 7 in, 2 out]
      }
      event "Save": Value Change {
        n11 = event-data() -> ()  [unwired: 1 in, 6 out]
        n12 = case shown="True" "Save" {
          tunnel: w25 -> [_ w26]
          frame False {
          }
          frame True {
            n13 = call "MCUS_STM.vi"("StateMachineSteps"=T4[] [{"main stm"=enum."Apply values", "data"=""}, {"main stm"=enum."Save", "data"=""}], "FNs"=enum16{"Back", "Front", "Replace"}."Back", "Queue in"=w26) -> ()  [unwired: 7 in, 2 out]
          }
        }
      }
      event "Open": Value Change {
        n14 = event-data() -> ()  [unwired: 1 in, 6 out]
        n15 = case shown="True" "Open" {
          tunnel: w30 -> [_ w31]
          frame False {
          }
          frame True {
            n16 = call "MCUS_STM.vi"("StateMachineSteps"=T4[] [{"main stm"=enum."Open", "data"=""}], "FNs"=enum16{"Back", "Front", "Replace"}."Back", "Queue in"=w31) -> ()  [unwired: 7 in, 2 out]
          }
        }
      }
      event "Reset": Value Change {
        n17 = event-data() -> ()  [unwired: 1 in, 6 out]
        n18 = case shown="True" "Reset" {
          tunnel: w35 -> [_ w36]
          frame False {
          }
          frame True {
            n19 = call "MCUS_STM.vi"("StateMachineSteps"=T4[] [{"main stm"=enum."Reset", "data"=""}], "FNs"=enum16{"Back", "Front", "Replace"}."Back", "Queue in"=w36) -> ()  [unwired: 7 in, 2 out]
          }
        }
      }
    }
  }
  n20 = while {
    tunnel: w7 -> [w48]
    tunnel: "Error In" -> [w44]
    tunnel: [w43] -> w5
    shift-right: [w42] -> w2
    shift-left: w4 -> [w40]
    shift-right: [w39] -> _
    shift-left: w4 -> [w39]
    stop <- w45 stop-if-true
    # "Loop (main)"
    n21 = Dequeue Element(queue=w48) -> (queue out=w41:refnum<queue>, element=w47:T4)  [unwired: 2 in, 2 out]
    n22 = Unbundle By Name(w47) -> ("main stm"=w46:T5)  [unwired: 1 out]
    n23 = case shown="\"Save\"" w46 {
      tunnel: w41 -> [_ _ _ _ _ _ w287 w304]
      tunnel: [_ _ FALSE FALSE TRUE _ _ _] -> w45
      tunnel: w44 -> [w50 w52 w55 w197 w269 _ _ _]
      tunnel: [w50 w52 w55 w197 w269 _ _ _] -> w43
      tunnel: [w49 w51 w53 w195 w267 w273 w289 w307] -> w42
      tunnel: w40 -> [w49 w51 w53 w149 w267 w273 w288 _]
      tunnel: w39 -> [_ _ _ _ _ _ _ w307]
      frame "idle", Default {
      }
      frame "_____ main_____ " {
      }
      frame "Init" {
        n24 = stacked-sequence {
          tunnel: w53 -> [_ w147]
          frame #0 {
            n25 = stacked-sequence {
              frame #0 {
                n26 = property on="Setting Path" class="Path"() -> ("Value"=w56:path)  [unwired: 2 in, 2 out]
                n27 = property on="Setting Path" class="Path"("Value"=w56) -> ()  [unwired: 2 in, 2 out]
              }
              frame #1 {
                # "Общие настройки"
                n28 = property on="Режим звонка тональный модем" class="Ring (strict)"() -> ("StringsAndValues[]"=w59:T8)  [unwired: 2 in, 2 out]
                n29 = property on="Алгоритм дозвона" class="Ring (strict)"() -> ("StringsAndValues[]"=w57:T8)  [unwired: 2 in, 2 out]
                n30 = property on="Аунтетификация" class="Ring (strict)"() -> ("StringsAndValues[]"=w66:T8)  [unwired: 2 in, 2 out]
                n31 = property on="Условия окружающей среды" class="Ring (strict)"() -> ("StringsAndValues[]"=w64:T8)  [unwired: 2 in, 2 out]
                n32 = property on="Источник питания" class="Ring (strict)"() -> ("StringsAndValues[]"=w65:T8)  [unwired: 2 in, 2 out]
                n33 = property on="Напряжение источника" class="Ring (strict)"() -> ("StringsAndValues[]"=w63:T8)  [unwired: 2 in, 2 out]
                n34 = property on="Режим звонка связь" class="Ring (strict)"() -> ("StringsAndValues[]"=w60:T8)  [unwired: 2 in, 2 out]
                n35 = property on="Сим карта" class="Ring (strict)"() -> ("StringsAndValues[]"=w68:T8)  [unwired: 2 in, 2 out]
                n36 = property on="Номер образца" class="Ring (strict)"() -> ("StringsAndValues[]"=w62:T8)  [unwired: 2 in, 2 out]
                n37 = property on="Номер испытания" class="Ring (strict)"() -> ("StringsAndValues[]"=w61:T8)  [unwired: 2 in, 2 out]
                n38 = property on="Количество итераций TM" class="DigNum (strict)"() -> ("Value"=w58:dbl)  [unwired: 2 in, 2 out]
                n39 = property on="Количество повторов измерений" class="DigNum (strict)"() -> ("Value"=w67:dbl)  [unwired: 2 in, 2 out]
                n40 = property on="Режим звонка тональный модем" class="Ring (strict)"("StringsAndValues[]"=w59) -> ()  [unwired: 2 in, 2 out]
                n41 = property on="Номер образца" class="Ring (strict)"("StringsAndValues[]"=w62) -> ()  [unwired: 2 in, 2 out]
                n42 = property on="Номер испытания" class="Ring (strict)"("StringsAndValues[]"=w61) -> ()  [unwired: 2 in, 2 out]
                n43 = property on="Сим карта" class="Ring (strict)"("StringsAndValues[]"=w68) -> ()  [unwired: 2 in, 2 out]
                n44 = property on="Алгоритм дозвона" class="Ring (strict)"("StringsAndValues[]"=w57) -> ()  [unwired: 2 in, 2 out]
                n45 = property on="Условия окружающей среды" class="Ring (strict)"("StringsAndValues[]"=w64) -> ()  [unwired: 2 in, 2 out]
                n46 = property on="Напряжение источника" class="Ring (strict)"("StringsAndValues[]"=w63) -> ()  [unwired: 2 in, 2 out]
                n47 = property on="Аунтетификация" class="Ring (strict)"("StringsAndValues[]"=w66) -> ()  [unwired: 2 in, 2 out]
                n48 = property on="Режим звонка связь" class="Ring (strict)"("StringsAndValues[]"=w60) -> ()  [unwired: 2 in, 2 out]
                n49 = property on="Количество повторов измерений" class="DigNum (strict)"("Value"=w67) -> ()  [unwired: 2 in, 2 out]
                n50 = property on="Количество итераций TM" class="DigNum (strict)"("Value"=w58) -> ()  [unwired: 2 in, 2 out]
                n51 = property on="Источник питания" class="Ring (strict)"("StringsAndValues[]"=w65) -> ()  [unwired: 2 in, 2 out]
              }
              frame #2 {
                # "Настройки модема по умолчанию"
                n52 = stacked-sequence {
                  frame #0 {
                    # "CMW500"
                    n53 = property on="VISA adress of CMW500" class="Str"() -> ("Value"=w69:string)  [unwired: 2 in, 2 out]
                    n54 = property on="Input attenuation" class="DigNum (strict)"() -> ("Value"=w70:dbl)  [unwired: 2 in, 2 out]
                    n55 = property on="Output attenuation" class="DigNum (strict)"() -> ("Value"=w71:dbl)  [unwired: 2 in, 2 out]
                    n56 = property on="VISA adress of CMW500" class="Str"("Value"=w69) -> ()  [unwired: 2 in, 2 out]
                    n57 = property on="Input attenuation" class="DigNum (strict)"("Value"=w70) -> ()  [unwired: 2 in, 2 out]
                    n58 = property on="Output attenuation" class="DigNum (strict)"("Value"=w71) -> ()  [unwired: 2 in, 2 out]
                  }
                  frame #1 {
                    # "GSM"
                    n59 = stacked-sequence {
                      frame #0 {
                        # "GSM Band/AWGN"
                        n60 = property on="GSM Band" class="Ring (strict)"() -> ("StringsAndValues[]"=w81:T8)  [unwired: 2 in, 2 out]
                        n61 = property on="UL C/I ratio" class="Ring (strict)"() -> ("StringsAndValues[]"=w74:T8)  [unwired: 2 in, 2 out]
                        n62 = property on="Codec" class="Ring (strict)"() -> ("StringsAndValues[]"=w78:T8)  [unwired: 2 in, 2 out]
                        n63 = property on="AWGN" class="Ring (strict)"() -> ("StringsAndValues[]"=w77:T8)  [unwired: 2 in, 2 out]
                        n64 = property on="GSM Fading" class="Ring (strict)"() -> ("StringsAndValues[]"=w75:T8)  [unwired: 2 in, 2 out]
                        n65 = property on="TCH Channel Power" class="DigNum (strict)"() -> ("Value"=w72:dbl)  [unwired: 2 in, 2 out]
                        n66 = property on="BCCH Channel Power" class="DigNum (strict)"() -> ("Value"=w73:dbl)  [unwired: 2 in, 2 out]
                        n67 = property on="BCCH Channel Number" class="DigNum (strict)"() -> ("Value"=w80:dbl)  [unwired: 2 in, 2 out]
                        n68 = property on="TCH Channel number" class="DigNum (strict)"() -> ("Value"=w79:dbl)  [unwired: 2 in, 2 out]
                        n69 = property on="snrRatioInDb" class="DigNum (strict)"() -> ("Value"=w76:dbl)  [unwired: 2 in, 2 out]
                        n70 = property on="GSM Band" class="Ring (strict)"("StringsAndValues[]"=w81) -> ()  [unwired: 2 in, 2 out]
                        n71 = property on="GSM Fading" class="Ring (strict)"("StringsAndValues[]"=w75) -> ()  [unwired: 2 in, 2 out]
                        n72 = property on="UL C/I ratio" class="Ring (strict)"("StringsAndValues[]"=w74) -> ()  [unwired: 2 in, 2 out]
                        n73 = property on="Codec" class="Ring (strict)"("StringsAndValues[]"=w78) -> ()  [unwired: 2 in, 2 out]
                        n74 = property on="AWGN" class="Ring (strict)"("StringsAndValues[]"=w77) -> ()  [unwired: 2 in, 2 out]
                        n75 = property on="BCCH Channel Number" class="DigNum (strict)"("Value"=w80) -> ()  [unwired: 2 in, 2 out]
                        n76 = property on="TCH Channel number" class="DigNum (strict)"("Value"=w79) -> ()  [unwired: 2 in, 2 out]
                        n77 = property on="snrRatioInDb" class="DigNum (strict)"("Value"=w76) -> ()  [unwired: 2 in, 2 out]
                        n78 = property on="TCH Channel Power" class="DigNum (strict)"("Value"=w72) -> ()  [unwired: 2 in, 2 out]
                        n79 = property on="BCCH Channel Power" class="DigNum (strict)"("Value"=w73) -> ()  [unwired: 2 in, 2 out]
                      }
                      frame #1 {
                        # "Custom network ID"
                        n80 = property on="MNC digit count" class="Ring (strict)"() -> ("StringsAndValues[]"=w90:T8)  [unwired: 2 in, 2 out]
                        n81 = property on="Use a custom network ID" class="Bool (strict)"() -> ("Value"=w93:bool)  [unwired: 2 in, 2 out]
                        n82 = property on="MCC (Mobile Country Code)" class="DigNum (strict)"() -> ("Value"=w92:dbl)  [unwired: 2 in, 2 out]
                        n83 = property on="MNC (Mobile Network Code)" class="DigNum (strict)"() -> ("Value"=w91:dbl)  [unwired: 2 in, 2 out]
                        n84 = property on="NCC (Network Color Code)" class="DigNum (strict)"() -> ("Value"=w89:dbl)  [unwired: 2 in, 2 out]
                        n85 = property on="BCC (Base station Color Code)" class="DigNum (strict)"() -> ("Value"=w88:dbl)  [unwired: 2 in, 2 out]
                        n86 = property on="RAC (Routing Area Code)" class="DigNum (strict)"() -> ("Value"=w87:dbl)  [unwired: 2 in, 2 out]
                        n87 = property on="Cell Identity" class="DigNum (strict)"() -> ("Value"=w86:dbl)  [unwired: 2 in, 2 out]
                        n88 = property on="Override UE ID" class="Bool (strict)"() -> ("Value"=w85:bool)  [unwired: 2 in, 2 out]
                        n89 = property on="MCC (UE Mobile Country Code)" class="DigNum (strict)"() -> ("Value"=w84:dbl)  [unwired: 2 in, 2 out]
                        n90 = property on="MNC (UE Mobile Network Code)" class="DigNum (strict)"() -> ("Value"=w83:dbl)  [unwired: 2 in, 2 out]
                        n91 = property on="MSIN (Mobile Subscription ID)" class="DigNum (strict)"() -> ("Value"=w82:dbl)  [unwired: 2 in, 2 out]
                        n92 = property on="Use a custom network ID" class="Bool (strict)"("Value"=w93) -> ()  [unwired: 2 in, 2 out]
                        n93 = property on="MCC (Mobile Country Code)" class="DigNum (strict)"("Value"=w92) -> ()  [unwired: 2 in, 2 out]
                        n94 = property on="MNC (Mobile Network Code)" class="DigNum (strict)"("Value"=w91) -> ()  [unwired: 2 in, 2 out]
                        n95 = property on="MNC digit count" class="Ring (strict)"("StringsAndValues[]"=w90) -> ()  [unwired: 2 in, 2 out]
                        n96 = property on="NCC (Network Color Code)" class="DigNum (strict)"("Value"=w89) -> ()  [unwired: 2 in, 2 out]
                        n97 = property on="BCC (Base station Color Code)" class="DigNum (strict)"("Value"=w88) -> ()  [unwired: 2 in, 2 out]
                        n98 = property on="RAC (Routing Area Code)" class="DigNum (strict)"("Value"=w87) -> ()  [unwired: 2 in, 2 out]
                        n99 = property on="Cell Identity" class="DigNum (strict)"("Value"=w86) -> ()  [unwired: 2 in, 2 out]
                        n100 = property on="Override UE ID" class="Bool (strict)"("Value"=w85) -> ()  [unwired: 2 in, 2 out]
                        n101 = property on="MCC (UE Mobile Country Code)" class="DigNum (strict)"("Value"=w84) -> ()  [unwired: 2 in, 2 out]
                        n102 = property on="MNC (UE Mobile Network Code)" class="DigNum (strict)"("Value"=w83) -> ()  [unwired: 2 in, 2 out]
                        n103 = property on="MSIN (Mobile Subscription ID)" class="DigNum (strict)"("Value"=w82) -> ()  [unwired: 2 in, 2 out]
                      }
                      frame #2 {
                        # "Call Release Type"
                        n104 = property on="Call Release Type" class="Ring (strict)"() -> ("StringsAndValues[]"=w94:T8)  [unwired: 2 in, 2 out]
                        n105 = property on="Call Release Type" class="Ring (strict)"("StringsAndValues[]"=w94) -> ()  [unwired: 2 in, 2 out]
                      }
                    }
                  }
                  frame #2 {
                    # "PSAP"
                    n106 = property on="InputScaleFactor" class="Ring (strict)"() -> ("StringsAndValues[]"=w100:T8)  [unwired: 2 in, 2 out]
                    n107 = property on="OutputScaleFactor" class="Ring (strict)"() -> ("StringsAndValues[]"=w99:T8)  [unwired: 2 in, 2 out]
                    n108 = property on="Scenario" class="Ring (strict)"() -> ("StringsAndValues[]"=w97:T8)  [unwired: 2 in, 2 out]
                    n109 = property on="AlAckBehavior" class="Ring (strict)"() -> ("StringsAndValues[]"=w96:T8)  [unwired: 2 in, 2 out]
                    n110 = property on="Post MSD wave file playback 3GPP  26.269 EU_DTMF_tones" class="Bool (strict)"() -> ("Value"=w98:bool)  [unwired: 2 in, 2 out]
                    n111 = property on="PSAP listens for PUSH" class="Bool (strict)"() -> ("Value"=w95:bool)  [unwired: 2 in, 2 out]
                    n112 = property on="InputScaleFactor" class="Ring (strict)"("StringsAndValues[]"=w100) -> ()  [unwired: 2 in, 2 out]
                    n113 = property on="OutputScaleFactor" class="Ring (strict)"("StringsAndValues[]"=w99) -> ()  [unwired: 2 in, 2 out]
                    n114 = property on="Post MSD wave file playback 3GPP  26.269 EU_DTMF_tones" class="Bool (strict)"("Value"=w98) -> ()  [unwired: 2 in, 2 out]
                    n115 = property on="Scenario" class="Ring (strict)"("StringsAndValues[]"=w97) -> ()  [unwired: 2 in, 2 out]
                    n116 = property on="AlAckBehavior" class="Ring (strict)"("StringsAndValues[]"=w96) -> ()  [unwired: 2 in, 2 out]
                    n117 = property on="PSAP listens for PUSH" class="Bool (strict)"("Value"=w95) -> ()  [unwired: 2 in, 2 out]
                  }
                }
              }
            }
          }
          frame #1 {
            n118 = Unbundle By Name(w147) -> ("Setting Path"=w103:path, "Номер образца"=w146:u16, "Номер испытания"=w145:u16, "Условия окружающей среды"=w144:u16, "Источник питания"=w143:u16, "Напряжение источника"=w142:u16, "Режим звонка связь"=w141:u16, "Аутентификация"=w138:u16, "Сим карта"=w136:u16, "Колличество повторов измерений"=w137:dbl, "Режим звонка тональный модем"=w140:u16, "Алгоритм дозвона"=w101:u16, "Количество итераций TM"=w139:dbl, "VISA adress of CMW500"=w135:string, "Input attenuation"=w134:dbl, "Output attenuation"=w133:dbl, "GSM Band"=w132:u16, "BCCH Channel Power"=w105:dbl, "TCH Channel Power"=w104:dbl, "BCCH Channel Number"=w102:dbl, "TCH Channel Number"=w131:dbl, "Codec"=w130:u16, "AWGN"=w129:u16, "snrRatioInDb"=w128:dbl, "GSM Fading"=w127:u16, "UL C/I ratio"=w126:u16, "Use a custom network ID"=w125:bool, "MCC (Mobile Country Code)"=w124:dbl, "MNC (Mobile Network Code)"=w123:dbl, "MNC digit count"=w122:u16, "NCC (Network Color Code)"=w121:dbl, "BCC (Base station Color Code)"=w120:dbl, "LAC (Location Area Code)"=w119:dbl, "RAC (Routing Area Code)"=w118:dbl, "Cell Identity"=w117:dbl, "Override UE ID"=w116:bool, "MCC (UE Mobile Country Code)"=w115:dbl, "MNC (UE Mobile Network Code)"=w114:dbl, "MSIN (Mobile Subscription ID)"=w113:dbl, "Call Release Type"=w112:u16, "InputScaleFactor"=w111:u16, "OutputScaleFactor"=w110:u16, "Post MSD wave file playback 3GPP  26.269 \nEU_DTMF_tones"=w109:bool, "Scenario"=w108:u16, "AlAckBehavior"=w107:u16, "PSAP listens for PUSH"=w106:bool)
            n119 = property on="Номер испытания" class="Ring (strict)"("Value"=w145) -> ()  [unwired: 2 in, 2 out]
            n120 = property on="Условия окружающей среды" class="Ring (strict)"("Value"=w144) -> ()  [unwired: 2 in, 2 out]
            n121 = property on="Источник питания" class="Ring (strict)"("Value"=w143) -> ()  [unwired: 2 in, 2 out]
            n122 = property on="Напряжение источника" class="Ring (strict)"("Value"=w142) -> ()  [unwired: 2 in, 2 out]
            n123 = property on="Режим звонка связь" class="Ring (strict)"("Value"=w141) -> ()  [unwired: 2 in, 2 out]
            n124 = property on="Аунтетификация" class="Ring (strict)"("Value"=w138) -> ()  [unwired: 2 in, 2 out]
            n125 = property on="Сим карта" class="Ring (strict)"("Value"=w136) -> ()  [unwired: 2 in, 2 out]
            n126 = property on="Количество повторов измерений" class="DigNum (strict)"("Value"=w137) -> ()  [unwired: 2 in, 2 out]
            n127 = property on="Режим звонка тональный модем" class="Ring (strict)"("Value"=w140) -> ()  [unwired: 2 in, 2 out]
            n128 = property on="Алгоритм дозвона" class="Ring (strict)"("Value"=w101) -> ()  [unwired: 2 in, 2 out]
            n129 = property on="Количество итераций TM" class="DigNum (strict)"("Value"=w139) -> ()  [unwired: 2 in, 2 out]
            n130 = property on="VISA adress of CMW500" class="Str"("Value"=w135) -> ()  [unwired: 2 in, 2 out]
            n131 = property on="Input attenuation" class="DigNum (strict)"("Value"=w134) -> ()  [unwired: 2 in, 2 out]
            n132 = property on="Output attenuation" class="DigNum (strict)"("Value"=w133) -> ()  [unwired: 2 in, 2 out]
            n133 = property on="GSM Band" class="Ring (strict)"("Value"=w132) -> ()  [unwired: 2 in, 2 out]
            n134 = property on="BCCH Channel Power" class="DigNum (strict)"("Value"=w105) -> ()  [unwired: 2 in, 2 out]
            n135 = property on="TCH Channel Power" class="DigNum (strict)"("Value"=w104) -> ()  [unwired: 2 in, 2 out]
            n136 = property on="BCCH Channel Number" class="DigNum (strict)"("Value"=w102) -> ()  [unwired: 2 in, 2 out]
            n137 = property on="TCH Channel number" class="DigNum (strict)"("Value"=w131) -> ()  [unwired: 2 in, 2 out]
            n138 = property on="Codec" class="Ring (strict)"("Value"=w130) -> ()  [unwired: 2 in, 2 out]
            n139 = property on="AWGN" class="Ring (strict)"("Value"=w129) -> ()  [unwired: 2 in, 2 out]
            n140 = property on="snrRatioInDb" class="DigNum (strict)"("Value"=w128) -> ()  [unwired: 2 in, 2 out]
            n141 = property on="GSM Fading" class="Ring (strict)"("Value"=w127) -> ()  [unwired: 2 in, 2 out]
            n142 = property on="UL C/I ratio" class="Ring (strict)"("Value"=w126) -> ()  [unwired: 2 in, 2 out]
            n143 = property on="Use a custom network ID" class="Bool (strict)"("Value"=w125) -> ()  [unwired: 2 in, 2 out]
            n144 = property on="MCC (Mobile Country Code)" class="DigNum (strict)"("Value"=w124) -> ()  [unwired: 2 in, 2 out]
            n145 = property on="MNC (Mobile Network Code)" class="DigNum (strict)"("Value"=w123) -> ()  [unwired: 2 in, 2 out]
            n146 = property on="MNC digit count" class="Ring (strict)"("Value"=w122) -> ()  [unwired: 2 in, 2 out]
            n147 = property on="NCC (Network Color Code)" class="DigNum (strict)"("Value"=w121) -> ()  [unwired: 2 in, 2 out]
            n148 = property on="BCC (Base station Color Code)" class="DigNum (strict)"("Value"=w120) -> ()  [unwired: 2 in, 2 out]
            n149 = property on="LAC (Location Area Code)" class="DigNum (strict)"("Value"=w119) -> ()  [unwired: 2 in, 2 out]
            n150 = property on="RAC (Routing Area Code)" class="DigNum (strict)"("Value"=w118) -> ()  [unwired: 2 in, 2 out]
            n151 = property on="Cell Identity" class="DigNum (strict)"("Value"=w117) -> ()  [unwired: 2 in, 2 out]
            n152 = property on="Override UE ID" class="Bool (strict)"("Value"=w116) -> ()  [unwired: 2 in, 2 out]
            n153 = property on="MCC (UE Mobile Country Code)" class="DigNum (strict)"("Value"=w115) -> ()  [unwired: 2 in, 2 out]
            n154 = property on="MNC (UE Mobile Network Code)" class="DigNum (strict)"("Value"=w114) -> ()  [unwired: 2 in, 2 out]
            n155 = property on="MSIN (Mobile Subscription ID)" class="DigNum (strict)"("Value"=w113) -> ()  [unwired: 2 in, 2 out]
            n156 = property on="Call Release Type" class="Ring (strict)"("Value"=w112) -> ()  [unwired: 2 in, 2 out]
            n157 = property on="InputScaleFactor" class="Ring (strict)"("Value"=w111) -> ()  [unwired: 2 in, 2 out]
            n158 = property on="OutputScaleFactor" class="Ring (strict)"("Value"=w110) -> ()  [unwired: 2 in, 2 out]
            n159 = property on="Post MSD wave file playback 3GPP  26.269 EU_DTMF_tones" class="Bool (strict)"("Value"=w109) -> ()  [unwired: 2 in, 2 out]
            n160 = property on="Scenario" class="Ring (strict)"("Value"=w108) -> ()  [unwired: 2 in, 2 out]
            n161 = property on="AlAckBehavior" class="Ring (strict)"("Value"=w107) -> ()  [unwired: 2 in, 2 out]
            n162 = property on="PSAP listens for PUSH" class="Bool (strict)"("Value"=w106) -> ()  [unwired: 2 in, 2 out]
            n163 = property on="Номер образца" class="Ring (strict)"("Value"=w146) -> ()  [unwired: 2 in, 2 out]
            n164 = property on="Setting Path" class="Path"("Value"=w103) -> ()  [unwired: 2 in, 2 out]
          }
        }
      }
      frame "Apply values" {
        n165 = flat-sequence {
          tunnel: ["InputScaleFactor"] -> w159
          tunnel: ["OutputScaleFactor"] -> w158
          tunnel: ["Post MSD wave file playback 3GPP  26.269 EU_DTMF_tones"] -> w157
          tunnel: ["Scenario"] -> w156
          tunnel: ["AlAckBehavior"] -> w155
          tunnel: ["PSAP listens for PUSH"] -> w154
          frame #0 {
            # "PSAP"
          }
        }
        n166 = flat-sequence {
          tunnel: [w227] -> w180
          tunnel: [w226] -> w153
          tunnel: [w225] -> w179
          tunnel: [w224] -> w178
          tunnel: [w223] -> w177
          tunnel: [w222] -> w176
          tunnel: [w221] -> w175
          tunnel: [w220] -> w174
          tunnel: [w219] -> w173
          tunnel: [w218] -> w172
          tunnel: [w217] -> w171
          tunnel: [w216] -> w170
          tunnel: [w215] -> w169
          tunnel: [w214] -> w168
          tunnel: [w213] -> w167
          tunnel: [w212] -> w166
          tunnel: [w211] -> w165
          tunnel: [w210] -> w164
          tunnel: [w209] -> w163
          tunnel: [w208] -> w162
          tunnel: [w207] -> w161
          tunnel: [w206] -> w160
          tunnel: [w205] -> w152
          tunnel: [w204] -> w151
          frame #0 {
            # "GSM"
            n167 = flat-sequence {
              tunnel: ["GSM Band"] -> w227
              tunnel: ["BCCH Channel Number"] -> w226
              tunnel: ["TCH Channel number"] -> w225
              tunnel: ["Codec"] -> w224
              tunnel: ["AWGN"] -> w223
              tunnel: ["snrRatioInDb"] -> w222
              tunnel: ["GSM Fading"] -> w221
              tunnel: ["UL C/I ratio"] -> w220
              tunnel: ["BCCH Channel Power"] -> w205
              tunnel: ["TCH Channel Power"] -> w204
              frame #0 {
                # "GSM Band/AWGN"
              }
            }
            n168 = flat-sequence {
              tunnel: ["Use a custom network ID"] -> w219
              tunnel: ["MCC (Mobile Country Code)"] -> w218
              tunnel: ["MNC (Mobile Network Code)"] -> w217
              tunnel: ["MNC digit count"] -> w216
              tunnel: ["NCC (Network Color Code)"] -> w215
              tunnel: ["BCC (Base station Color Code)"] -> w214
              tunnel: ["LAC (Location Area Code)"] -> w213
              tunnel: ["RAC (Routing Area Code)"] -> w212
              tunnel: ["Cell Identity"] -> w211
              tunnel: ["Override UE ID"] -> w210
              tunnel: ["MCC (UE Mobile Country Code)"] -> w209
              tunnel: ["MNC (UE Mobile Network Code)"] -> w208
              tunnel: ["MSIN (Mobile Subscription ID)"] -> w207
              frame #0 {
                # "Custom network ID"
              }
            }
            n169 = flat-sequence {
              tunnel: ["Call Release Type"] -> w206
              frame #0 {
                # "Call Release Type"
              }
            }
          }
        }
        n170 = flat-sequence {
          tunnel: ["VISA adress of CMW500"] -> w186
          tunnel: ["Input attenuation"] -> w185
          tunnel: ["Output attenuation"] -> w184
          frame #0 {
            # "CMW500"
          }
        }
        n171 = flat-sequence {
          tunnel: ["Номер образца"] -> w194
          tunnel: ["Номер испытания"] -> w193
          tunnel: ["Условия окружающей среды"] -> w192
          tunnel: ["Источник питания"] -> w191
          tunnel: ["Напряжение источника"] -> w190
          tunnel: ["Режим звонка связь"] -> w189
          tunnel: ["Аунтетификация"] -> w188
          tunnel: ["Сим карта"] -> w187
          tunnel: ["Количество повторов измерений"] -> w183
          tunnel: ["Режим звонка тональный модем"] -> w182
          tunnel: ["Количество итераций TM"] -> w181
          tunnel: ["Алгоритм дозвона"] -> w148
          frame #0 {
            # "Общие настройки"
          }
        }
        n172 = Bundle By Name(cluster=w149, "Setting Path"="Setting Path", "Номер образца"=w194, "Номер испытания"=w193, "Условия окружающей среды"=w192, "Источник питания"=w191, "Напряжение источника"=w190, "Режим звонка связь"=w189, "Аутентификация"=w188, "Сим карта"=w187, "Колличество повторов измерений"=w183, "Режим звонка тональный модем"=w182, "Алгоритм дозвона"=w148, "Количество итераций TM"=w181, "VISA adress of CMW500"=w186, "Input attenuation"=w185, "Output attenuation"=w184, "GSM Band"=w180, "BCCH Channel Power"=w152, "TCH Channel Power"=w151, "BCCH Channel Number"=w153, "TCH Channel Number"=w179, "Codec"=w178, "AWGN"=w177, "snrRatioInDb"=w176, "GSM Fading"=w175, "UL C/I ratio"=w174, "Use a custom network ID"=w173, "MCC (Mobile Country Code)"=w172, "MNC (Mobile Network Code)"=w171, "MNC digit count"=w170, "NCC (Network Color Code)"=w169, "BCC (Base station Color Code)"=w168, "LAC (Location Area Code)"=w167, "RAC (Routing Area Code)"=w166, "Cell Identity"=w165, "Override UE ID"=w164, "MCC (UE Mobile Country Code)"=w163, "MNC (UE Mobile Network Code)"=w162, "MSIN (Mobile Subscription ID)"=w161, "Call Release Type"=w160, "InputScaleFactor"=w159, "OutputScaleFactor"=w158, "Post MSD wave file playback 3GPP  26.269 \nEU_DTMF_tones"=w157, "Scenario"=w156, "AlAckBehavior"=w155, "PSAP listens for PUSH"=w154) -> (w195:T6)
      }
      frame "Stop" {
      }
      frame "Save" {
        n173 = property on="Setting Path" class="Path"() -> ("Value"=w272:path)  [unwired: 2 in, 2 out]
        n174 = Strip Path(path=w272) -> (stripped path=w271:path, name=w270:string)
        n175 = call "File Dialog"("start path"=w271, "default name"=w270, "pattern (all files)"="*.cnf", "pattern label"="cnf file") -> ("selected path"=w275:path, "error out"=w274:errorcluster)  [unwired: 8 in, 2 out]
        n176 = case shown="No Error" w274 {
          tunnel: w273 -> [w280 _]
          tunnel: w275 -> [w279 _]
          frame No Error {
            n177 = Bundle By Name(cluster=w280, "Setting Path"=w279) -> (w278:T6)
            n178 = call <vilib>:"Flatten To JSON String.vi"("Numeric Extensions (F)"=FALSE, "Variant"=w278) -> ("JSON String"=w282:string)  [unwired: 8 in, 1 out]
            n179 = call "MFLI_File_write.vi"("String"=w282, "operation (0:open)"=T7."replace or create with confirmation", "selected path"=w279) -> ()  [unwired: 7 in, 2 out]
            n180 = property on="Setting Path" class="Path"("Value"=w279) -> ()  [unwired: 2 in, 2 out]
          }
          frame Error {
          }
        }
      }
      frame "Open" {
        n181 = property on="Setting Path" class="Path"() -> ("Value"=w286:path)  [unwired: 2 in, 2 out]
        n182 = Strip Path(path=w286) -> (stripped path=w284:path, name=w285:string)
        n183 = call "File Dialog2"("start path"=w284, "default name"=w285, "pattern (all files)"="*.cnf", "pattern label"="cnf file") -> ("selected path"=w291:path, "error out"=w290:errorcluster)  [unwired: 8 in, 2 out]
        n184 = case shown="No Error" w290 {
          tunnel: w291 -> [w294 _]
          tunnel: w287 -> [w300 _]
          tunnel: w288 -> [w298 w303]
          tunnel: [w295 w303] -> w289
          frame No Error {
            n185 = call "MFLI_File_read.vi"("Project script or program"=w294) -> ("String"=w299:string)  [unwired: 9 in, 1 out]
            n186 = call <vilib>:"Unflatten From JSON String.vi"("Type and Defaults"=w298, "JSON String"=w299) -> ("Variant"=w297:variant)  [unwired: 8 in, 1 out]
            n187 = Variant To Data(type=w298, Variant=w297) -> (data=w296:T6)  [unwired: 1 in, 1 out]
            n188 = Bundle By Name(cluster=w296, "Setting Path"=w294) -> (w295:T6)
            n189 = property on="Setting Path" class="Path"("Value"=w294) -> ()  [unwired: 2 in, 2 out]
            n190 = call "MCUS_STM.vi"("StateMachineSteps"=T4[] [{"main stm"=enum."Init", "data"=""}], "FNs"=enum16{"Back", "Front", "Replace"}."Back", "Queue in"=w300) -> ()  [unwired: 7 in, 2 out]
          }
          frame Error {
          }
        }
      }
      frame "Reset" {
        n191 = call "MCUS_STM.vi"("StateMachineSteps"=T4[] [{"main stm"=enum."Init", "data"=""}], "FNs"=enum16{"Back", "Front", "Replace"}."Back", "Queue in"=w304) -> ()  [unwired: 7 in, 2 out]
      }
    }
  }
  "Error Out" <- w5
  n192 = Bundle By Name(cluster="CSMinfo in", "Окно с настройками"=w2) -> (→"CSMinfo out":T3)
